vi "CurlingRobotforThrowingSTD.vi"() -> ()   [LabVIEW 2018]
uses:
  <vilib>/myRIO/Instrument Drivers/Onboard IO/DIO/typedefs/DIO Reference.ctl
  <vilib>/myRIO/Common/Instrument Driver Framework/Utilities/typedefs/myRIO Generic Hardware Reference.ctl
  <vilib>/myRIO/Common/Instrument Driver Framework/Utilities/typedefs/Hardware Version Enum.ctl
  <vilib>/myRIO/Common/Instrument Driver Framework/Utilities/typedefs/myRIO v1.0 Reference.ctl
  <vilib>/myRIO/Common/Instrument Driver Framework/Utilities/typedefs/Generic FPGA Reference.ctl
  <vilib>/myRIO/Common/Instrument Driver Framework/myRIO v1.0/DIO/typedefs/DIO Channels List.ctl
  <vilib>/myRIO/Common/Instrument Driver Framework/myRIO v1.0/DIO/typedefs/DIO Channels Enum.ctl
  <vilib>/userdefined/High Color/nirio_resource_hc.ctl
  <vilib>/myRIO/Instrument Drivers/Onboard IO/AO/typedefs/AO Reference.ctl
  <vilib>/myRIO/Common/Instrument Driver Framework/myRIO v1.0/AO/typedefs/AO Channels List.ctl
  <vilib>/myRIO/Common/Instrument Driver Framework/myRIO v1.0/AO/typedefs/AO Channels Enum.ctl
  <vilib>/myRIO/Common/Instrument Driver Framework/Utilities/typedefs/Analog Scaling Constants List.ctl
  <vilib>/myRIO/Common/Instrument Driver Framework/Utilities/typedefs/Analog Scaling Constants.ctl
  <vilib>/myRIO/Instrument Drivers/Onboard IO/I2C/typedefs/I2C User Configuration.ctl
  <vilib>/myRIO/Instrument Drivers/Onboard IO/I2C/typedefs/I2C Transfer Rate.ctl
  <vilib>/Platform/TimedLoop/XDataNode/timing_clust.ctl
  <vilib>/Platform/TimedLoop/XDataNode/nitl_modes.ctl
  <vilib>/Platform/TimedLoop/XDataNode/wakeup.ctl
  <vilib>/myRIO/Instrument Drivers/Onboard Devices/Accelerometer/typedefs/Accelerometer Reference.ctl
  <vilib>/myRIO/Common/Instrument Driver Framework/myRIO v1.0/Accelerometer/typedefs/Accelerometer Channels List.ctl
  <vilib>/myRIO/Common/Instrument Driver Framework/myRIO v1.0/Accelerometer/typedefs/Accelerometer Channels Enum.ctl
  <vilib>/myRIO/Common/Instrument Driver Framework/myRIO v1.0/Encoder/typedefs/Encoder Signal Mode.ctl
  <vilib>/myRIO/Instrument Drivers/Onboard IO/Encoder/typedefs/Encoder Reference.ctl
  <vilib>/myRIO/Common/Instrument Driver Framework/myRIO v1.0/Encoder/typedefs/Encoder Channels Enum.ctl
  <vilib>/myRIO/Common/Instrument Driver Framework/myRIO v1.0/Encoder/typedefs/Encoder Configuration v1.0.ctl
  <vilib>/myRIO/Common/Instrument Driver Framework/Utilities/vis/Is FPGA Ref Available.vi
  <vilib>/myRIO/Common/Instrument Driver Framework/myRIO v1.0/DIO/vis/myRIO v1.1 Open DIO.vi
  <vilib>/myRIO/Common/Instrument Driver Framework/myRIO v1.0/AO/vis/myRIO v1.1 Open AO.vi
  <vilib>/myRIO/Common/Instrument Driver Framework/myRIO v1.0/Accelerometer/vis/myRIO v1.1 Open Accelerometer.vi
  <vilib>/myRIO/Instrument Drivers/Onboard Devices/Accelerometer/vis/Read.vi
  <vilib>/myRIO/Common/Instrument Driver Framework/myRIO v1.0/Encoder/vis/myRIO v1.1 Open Encoder.vi
  <vilib>/myRIO/Instrument Drivers/Onboard IO/Encoder/vis/Read.vi
  <vilib>/myRIO/Common/Instrument Driver Framework/Utilities/vis/Validate Channels.vi
  <vilib>/myRIO/Common/Instrument Driver Framework/myRIO v1.0/DIO/vis/myRIO v1.0 Reserve DIO.vi
  <vilib>/myRIO/Common/Instrument Driver Framework/myRIO v1.0/AO/vis/myRIO v1.0 Reserve AO.vi
  <vilib>/myRIO/Common/Instrument Driver Framework/myRIO v1.0/Accelerometer/vis/myRIO v1.0 Reserve Accelerometer.vi
  <vilib>/myRIO/Common/Instrument Driver Framework/myRIO v1.0/I2C/vis/myRIO v1.1 Open I2C.vi
  <vilib>/myRIO/Common/Instrument Driver Framework/myRIO v1.0/Encoder/vis/myRIO v1.0 Reserve Encoder.vi
  <vilib>/myRIO/Common/Instrument Driver Framework/myRIO v1.0/UART/vis/myRIO v1.0 Close UART.vi
  <vilib>/myRIO/Common/Instrument Driver Framework/myRIO v1.0/Resource Manager/vis/myRIO v1.0 Reserve Channel List.vi
  <vilib>/myRIO/Common/Instrument Driver Framework/myRIO v1.0/DIO/vis/myRIO v1.0 Build MUX Configuration DIO.vi
  <vilib>/myRIO/Common/Instrument Driver Framework/myRIO v1.0/AO/vis/myRIO v1.0 Build MUX Configuration AO.vi
  <vilib>/myRIO/Common/Instrument Driver Framework/myRIO v1.0/Accelerometer/vis/myRIO v1.0 Build MUX Configuration Accelerometer.vi
  <vilib>/myRIO/Common/Instrument Driver Framework/myRIO v1.0/I2C/vis/myRIO v1.0 Reserve I2C.vi
  <vilib>/myRIO/Common/Instrument Driver Framework/myRIO v1.0/Encoder/vis/myRIO v1.0 Build MUX Configuration Encoder.vi
  <vilib>/myRIO/Common/Instrument Driver Framework/myRIO v1.0/Resource Manager/vis/myRIO v1.0 Reserve Channel.vi
  <vilib>/myRIO/Common/Instrument Driver Framework/myRIO v1.0/Resource Manager/vis/myRIO v1.0 Unreserve Channel.vi
  <vilib>/myRIO/Common/Instrument Driver Framework/myRIO v1.0/Resource Manager/vis/myRIO v1.0 Create Configuration List.vi
  <vilib>/myRIO/Common/Instrument Driver Framework/myRIO v1.0/I2C/vis/myRIO v1.0 Build MUX Configuration I2C.vi
  <vilib>/myRIO/Common/Instrument Driver Framework/myRIO v1.0/Resource Manager/vis/myRIO v1.0 Build Mutex Name.vi
  <vilib>/Instr/_visa.llb/VISA Configure Serial Port (Instr).vi
  <vilib>/Utility/VariantDataType/GetNumericInfo.vi
  <vilib>/Utility/error.llb/Error Cluster From Error Code.vi
  <vilib>/myRIO/Common/Instrument Driver Framework/myRIO v1.0/myRIO v1.1 Open.vi
  <vilib>/myRIO/Common/Instrument Driver Framework/Utilities/vis/IO Manager.vi
  <vilib>/myRIO/Common/Instrument Driver Framework/Utilities/vis/Configuration Manager.vi
  <vilib>/myRIO/Common/Instrument Driver Framework/myRIO v1.0/Resource Manager/vis/myRIO v1.0 Configure IO.vi
  <vilib>/myRIO/Common/Instrument Driver Framework/myRIO v1.0/myRIO v1.0 Close.vi
  <vilib>/myRIO/Common/Instrument Driver Framework/myRIO v1.0/DIO/vis/myRIO v1.0 Write DIO.vi
  <vilib>/myRIO/Common/Instrument Driver Framework/myRIO v1.0/AO/vis/myRIO v1.0 Get Scaling Constants AO.vi
  <vilib>/myRIO/Common/Instrument Driver Framework/myRIO v1.0/AO/vis/myRIO v1.0 Write AO.vi
  <vilib>/myRIO/Common/Instrument Driver Framework/myRIO v1.0/I2C/vis/myRIO v1.0 Configure I2C.vi
  <vilib>/myRIO/Common/Instrument Driver Framework/myRIO v1.0/I2C/vis/myRIO v1.0 Write I2C.vi
  <vilib>/myRIO/Common/Instrument Driver Framework/myRIO v1.0/Encoder/vis/myRIO v1.0 Configure Encoder.vi
  <vilib>/myRIO/Common/Instrument Driver Framework/myRIO v1.0/Encoder/vis/myRIO v1.0 Read Encoder.vi
  <vilib>/myRIO/Common/Instrument Driver Framework/myRIO v1.0/I2C/vis/myRIO v1.0 Read I2C.vi
  <vilib>/myRIO/Common/Instrument Driver Framework/Utilities/vis/FPGA Ref Manager.vi
  <vilib>/myRIO/Common/Instrument Driver Framework/myRIO v1.0/myRIO v1.0 Reset FPGA.vi
  <vilib>/myRIO/Common/Instrument Driver Framework/myRIO v1.0/IRQ/vis/myRIO v1.0 IRQ Info FGV.vi
  <vilib>/myRIO/Common/Instrument Driver Framework/myRIO v1.0/IRQ/vis/myRIO v1.0 Timer IRQ Info FGV.vi
  <vilib>/myRIO/Common/Instrument Driver Framework/myRIO v1.0/IRQ/vis/myRIO v1.0 ISR Agent.vi
  <vilib>/myRIO/Common/Instrument Driver Framework/myRIO v1.0/Accelerometer/vis/myRIO v1.0 Get Scaling Constant Accelerometer.vi
  <vilib>/myRIO/Common/Instrument Driver Framework/myRIO v1.0/Accelerometer/vis/myRIO v1.0 Read Accelerometer.vi
  <vilib>/myRIO/Express VI/Onboard IO/DO/DO Express VI.xnode
  <vilib>/myRIO/Instrument Drivers/Onboard IO/DIO/vis/myRIO DIO Open.xnode
  <vilib>/myRIO/Express VI/Onboard IO/AO/AO Express VI.xnode
  <vilib>/myRIO/Instrument Drivers/Onboard IO/AO/vis/myRIO AO Open.xnode
  <vilib>/Platform/TimedLoop/XDataNode/XDataNode.xnode
  <vilib>/myRIO/Express VI/Onboard IO/Encoder/Encoder Express VI.xnode
  <vilib>/myRIO/Instrument Drivers/Onboard IO/Encoder/vis/myRIO Encoder Open.xnode
  <vilib>/myRIO/Common/Instrument Driver Framework/myRIO v1.0/Encoder/typedefs/Encoder Count Direction Enum.ctl
  <vilib>/myRIO/Express VI/Onboard Devices/Accelerometer/Accelerometer Express VI.xnode
  <vilib>/myRIO/Instrument Drivers/Onboard Devices/Accelerometer/vis/myRIO Accelerometer Open.xnode
  <vilib>/Platform/TimedLoop/XDataNode/XDNodeRunTimeDep.lvlib
  <vilib>/myRIO/Instrument Drivers/Onboard IO/I2C/I2C.lvlib
  <vilib>/myRIO/Instrument Drivers/Utilities/Utilities.lvlib
  <vilib>/myRIO/Instrument Drivers/Onboard IO/Encoder/Encoder.lvlib
  <vilib>/myRIO/Instrument Drivers/Onboard IO/DIO/DIO.lvlib
  <vilib>/myRIO/Instrument Drivers/Onboard IO/AO/AO.lvlib
  <vilib>/myRIO/Instrument Drivers/Onboard Devices/Accelerometer/Accelerometer.lvlib
panel:
  out "DEn":bool
  out "StEn":bool
  out "RearEn":i16
  out "Readyon":bool
  out "YRRef":dbl
  out "YRRefOn":dbl
  out "RotFB":dbl
  out "RotFF":dbl
  out "IniSteerCmd":dbl=-0.08438764299664774
  in  "deg/Volt":dbl=2.8
  in  "SteerOri":dbl=391.05
  in  "StRefCut":dbl=1.0
  out "Tq_Steer":dbl=5.4e-323
  out "ori_phi":dbl(graph)=352.282379
  in  "SaveReset":bool
  in  "file create":bool
  out "File create":i32
  out "write":bool
  out "data innter":i32
  out "reset":bool
  out "Numeric Control":i32
  out "DriveMode":dbl(graph)=5.0
  out "PhiErr":dbl=-0.07207549693756998
  in  "LimStopErrVel":dbl=1.1
  in  "Cut_StopErr":dbl=3.0
  in  "KpStopError":dbl=10.0 format="%#_13g"
  in  "Ome_FB_Ratelimit(off)":bool=TRUE
  in  "Rear_scale":dbl=1.5 format="%#_13g"
  in  "FFOn":bool=TRUE
  in  "scale_Ang_steer/ 2":dbl=1.0 format="%#_13g"
  out "Tq_vel":cluster{dbl, dbl, "MinW":dbl}(graph)={-2.87e-322, -2.87e-322, "MinW"=2e-323} caption="CompareVel"
  in  "ShiftVelcrit":dbl=0.93 format="%#_13g"
  out "Ang":cluster{dbl, "y":dbl, dbl}(graph)
  out "AngError":dbl=2.6668637993124005
  out "tq":i32=5
  out "kvh":i32=501
  in  "No SRC(off)":bool=TRUE
  in  "Anti_wind":bool
  out "Wind_E":dbl
  in  "K_antiwind":dbl=0.5
  in  "criteria ang1":dbl=0.07
  in  "criteria ang2":dbl=2.0
  in  "ini_phi_2":dbl=5.0
  in  "ini_phi_1":dbl=1.5
  in  "DriveStart_manual":bool
  out "Driving":bool
  out "Ome_R":dbl=1.8e-322
  out "Ome_L":dbl=1.8e-322
  out "AngNowFB":dbl=-0.8036161356018248
  in  "scale_Ang_steer/":dbl=1.5 format="%#_13g"
  in  "Mode4_manual\n(get now ang)":bool
  in  "YR*_Off(manual)":bool=TRUE
  in  "From_SBC_DOB":bool
  in  "V*manualn":dbl=0.8
  in  "AutoSBCOn":bool=TRUE
  in  "Angle*_manual":dbl
  out "Time_int":i32=2781129
  in  "Steeing_Tq*_limit":dbl=5.0
  in  "YawConton":bool
  in  "Rear_DriveE":bool
  in  "Drive_Enable":bool
  in  "Rear_steerEnable":bool
  in  "Front enable":bool
  in  "Kt_longi":dbl=0.12
  in  "B_FF_R_wh":dbl=0.008
  in  "J_FF_R_wh":dbl=0.05
  in  "right wheel FF_cut 2":dbl=8.0
  in  "ylimit":dbl=0.2 format="%#_13g"
  out "Ome_ref":dbl
  in  "sigma_rate":dbl=0.0008 format="%#_13g"
  out "Ome_rear":dbl=-1.8e-322
  out "V+yS":dbl=2e-323
  out "VwRef":dbl=2e-323
  out "V+yV":dbl=2e-323
  out "y*(Ki+Kp)":dbl=-2.5e-323
  out "Ki_y":dbl
  out "Kp_y":dbl=-2.5e-323
  out "Vref":dbl
  in  "Vw*limitby_sigma":dbl=1.0 format="%#_13g"
  in  "Vel_treshold":dbl=0.6 format="%#_13g"
  in  "(1+y)_change":dbl=1.0 format="%#_13g"
  in  "Kp_V_cont 2":dbl=1.3
  in  "Ki_V_cont":dbl
  out "Sigmafor V+ySigma=Vw":dbl
  in  "Ki_wheel\nomega_cont":dbl
  in  "Kp_wheelomega_Cont":dbl=1.9
  out "Tq_cmd_R":dbl=-2.87e-322
  out "Tq_cmd_L":dbl=-2.87e-322
  in  "Tq limit[V]":dbl=10.0
  out "Vel_Robot":dbl=2e-323
  in  "Wheelvel_ratelimit cut":dbl=20.0
  in  "wheelV_ratelimit":dbl=0.001
  out "th_steer":dbl=0.11066568835903608
  in  "Enc_steer":bool
  out "l_rear":dbl=0.1917516891011395
  in  "Enc_set 0":bool
  out "l_L 2":dbl=0.1944940376883356
  out "l_R 2":dbl=0.14254976665663685
  in  "Tq_stop":dbl=-3.0 format="%#_13g"
  out "back stop":bool
  out "back driving act":bool
  in  "Desire back dist":dbl=2.5
  out "Back driving time":dbl=47.62300000000005
  in  "nowphi_in":dbl
  out "dist_avr":dbl=0.14254976665663685
  in  "ref_LFP_cut":dbl=10.0
  in  "ang_compensate":dbl
  in  "Bm_rot FF":dbl=0.1
  in  "Jm_rotFF":dbl=0.1
  in  "gyro scale":dbl=0.3
  out "delta_ang_memo":dbl
  out "fine_tunning":sgl=1.0
  out "nowphi":dbl
  in  "Stop":bool
  out "Data":string
  out "*(타입 *) &x":T1={"header"=43520, "type"=10, "data0"=5.0, "data1"=390.6329}
  out "driveONoFF":dbl format="%#_13g"
  out "DriveMODE":dbl=5.0 format="%#_13g"
  out "SteerAng":dbl=390.6329040527344 format="%#_13g"
  out "Target_V":dbl=2.3801119327545166 format="%#_13g"
  out "angle":dbl=2.4951019287109375 format="%#_13g"
  in  "Server Closed":string="The server VI closed the connection."
  in  "Stop Button":bool
  in  "phi_target":dbl
  in  "Kt_rot":dbl=0.093 format="%#_13g"
  out "AngNowCmd":dbl=-0.8756916325393947
  in  "PD_cut_rot 2":dbl=10.0
  in  "Kp_rot 3":dbl=0.0005
  in  "Kd_rot 4":dbl=0.0001
  out "ang_bias remover":dbl=0.8036191995518251
  out "Abs angle or gyro":dbl=352.282379
  in  "abs gy stop Button":bool
  in  "ratelimit band":dbl=0.0009
  in  "ratelimit cut":dbl=30.0
  in  "yaw_ratelimit":dbl=0.003
  out "time_now":u32=3177835
  out "Tq ang in":dbl=8e-323
  out "DOB FB":dbl=-0.0
  out "GyroFB":dbl
  in  "gy_offset_remover cutoff":dbl=0.05
  in  "Kd_rot 3":dbl=0.001
  in  "Kp_rot 2":dbl=0.005
  in  "PD_cut_rot":dbl=13.0
  in  "FF_cut":dbl=5.0
  in  "DOB_FB_cut":dbl=13.0
  in  "Bm_rot":dbl=0.1
  in  "Jm_rot":dbl=0.15
  in  "Vel_cut":dbl=25.0
  out "Z rate":i16=253
  in  "[main loop]":bool
  out "Tq_cmd_Rear":dbl=2.57e-322
  # "manual Driving"
  # "manual Driving and Auto from SBC selection"
  # "Auto Driving"
  # "Initial"
  # "Yaw ref"
  # "longi vel cmd"
  # "Output"
  # "wheel_vel_ratelimeter"
  # "Longi vel control"
  # "SRC"
  # "Anti-wind"
  # "Yaw control"
  # "Yaw  rate control"
  # "Dimension values"
  # "Yaw  rate control"
  # "Auto back"
  # "Fine turnning"
  # "anti windup"
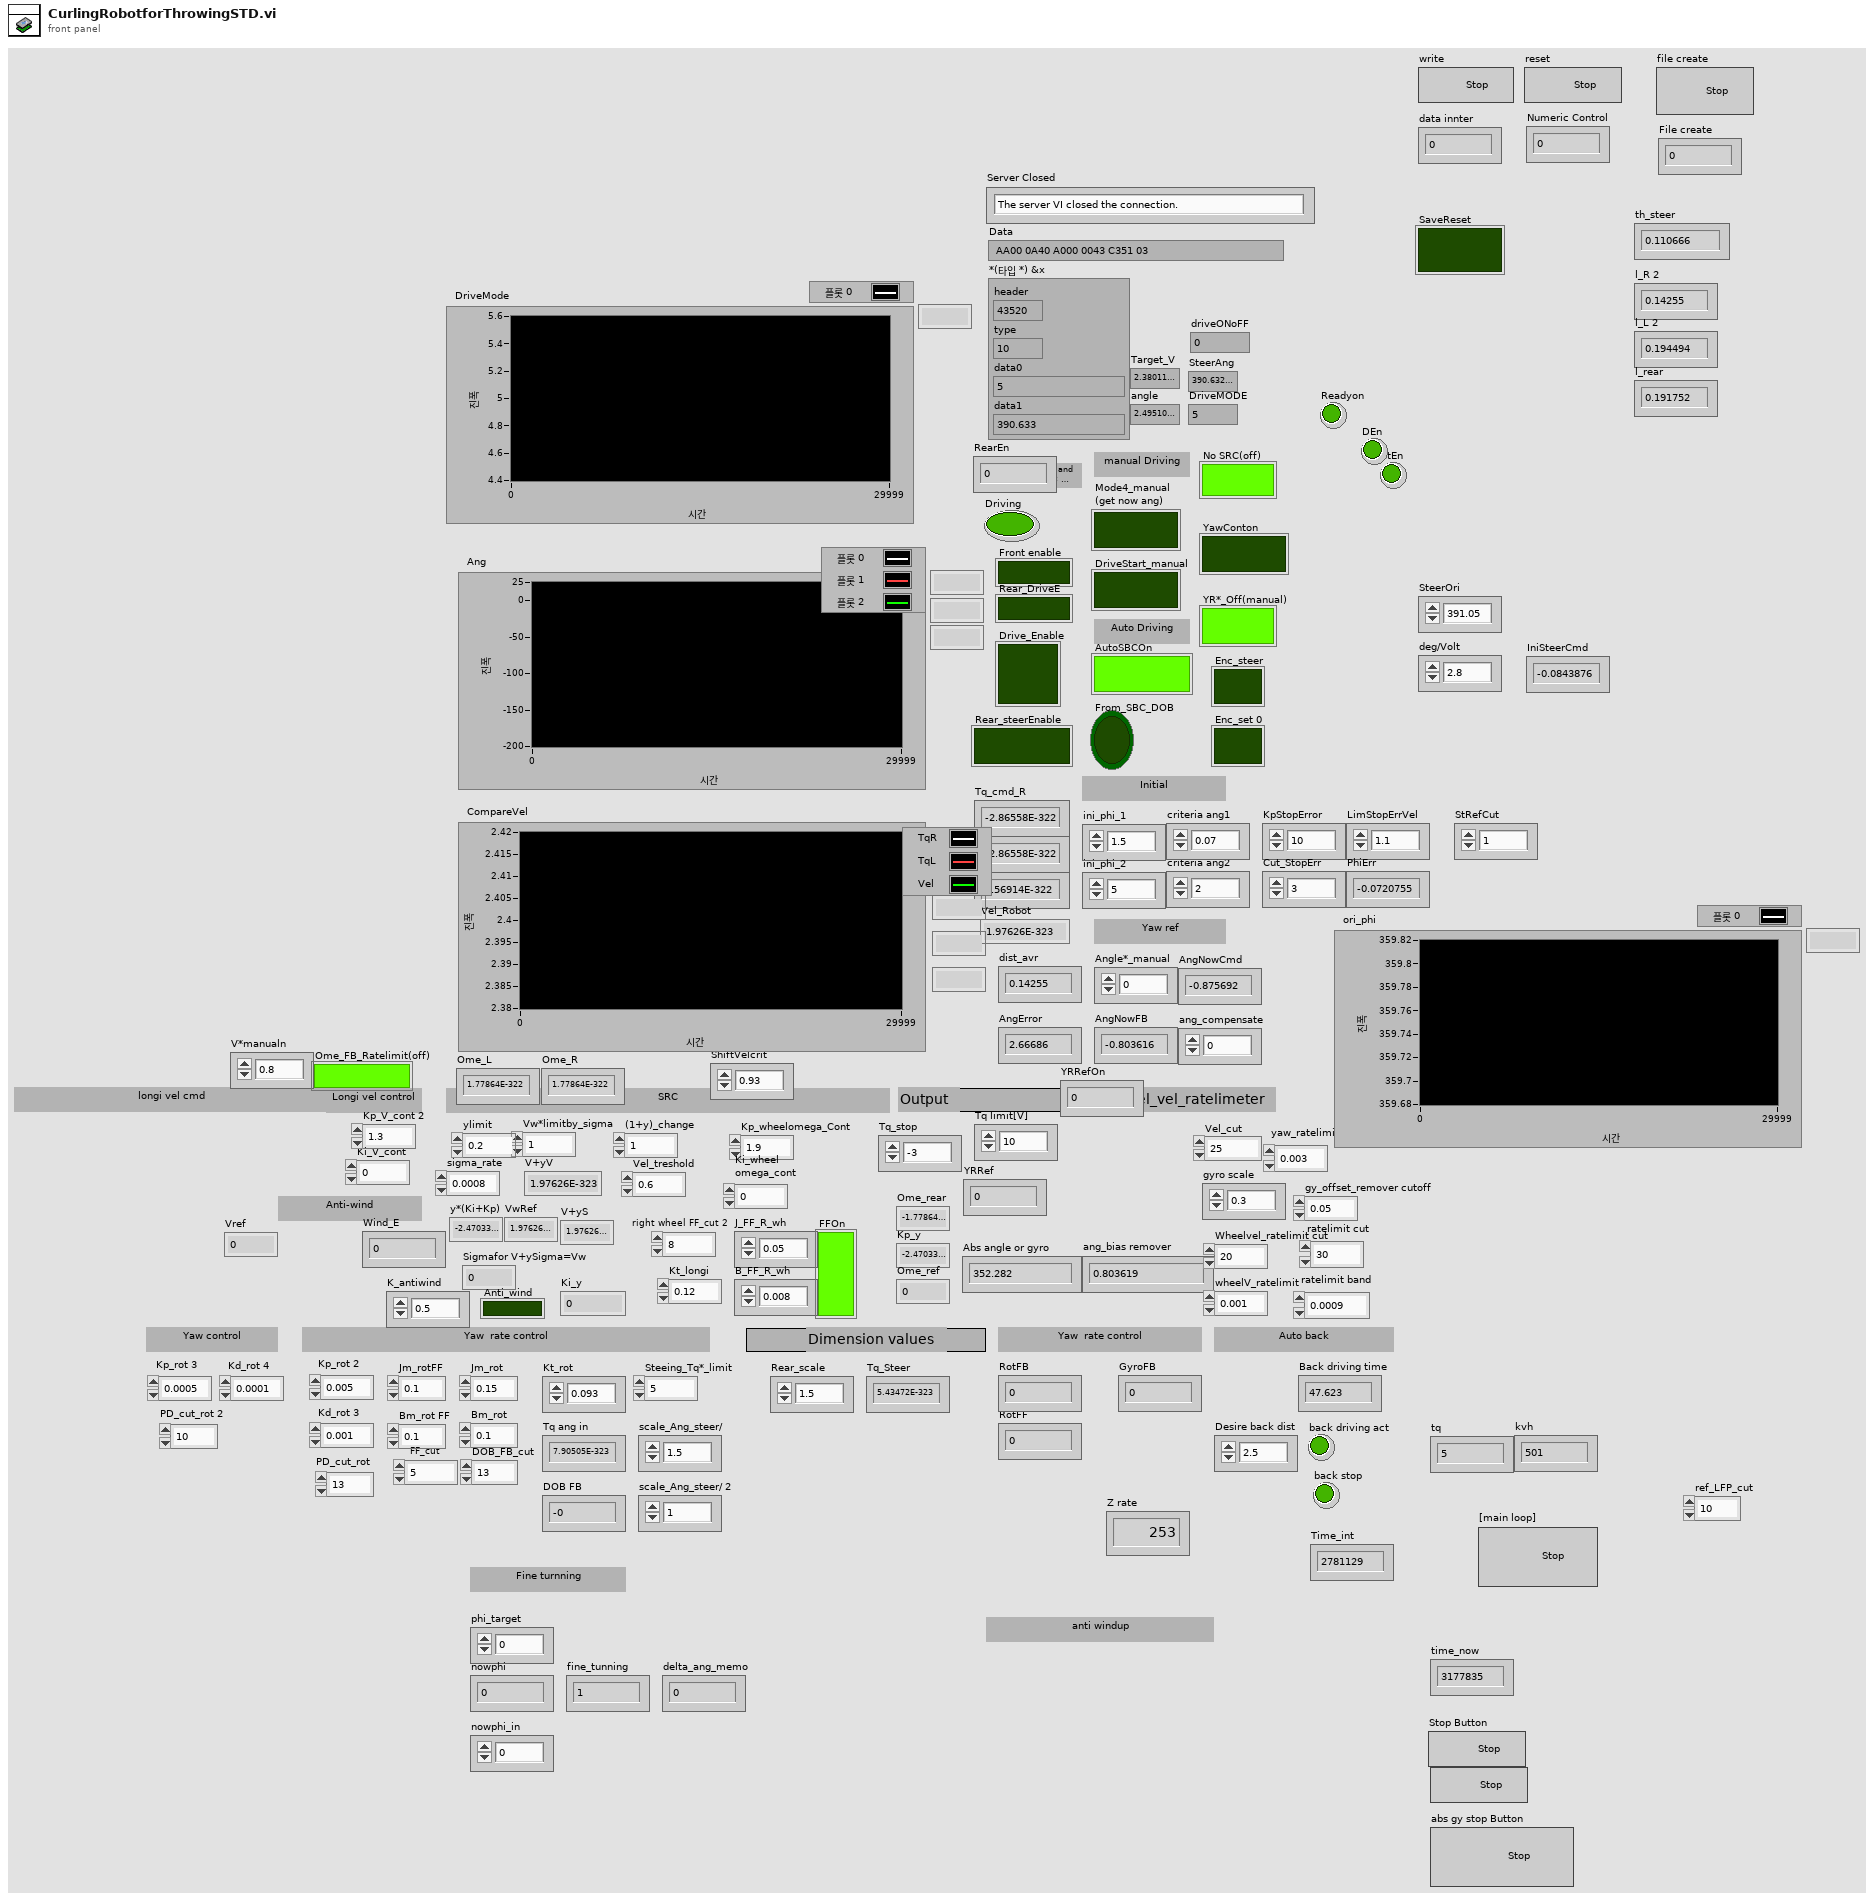
[diagram p1: front panel]
types:
  T1 = cluster{"header":u16, "type":u8, "data0":sgl, "data1":sgl}
  T2 = typedef "DIO.lvlib/DIO Reference.ctl" = cluster{"myRIO Reference":T3, "DIO Channels List":T7}
  T3 = typedef "myRIO Generic Hardware Reference.ctl" = cluster{"myRIO Model":T4, "myRIO Hardware Reference":T5}
  T4 = typedef "Hardware Version Enum.ctl" = enum16{"Unknown", "myRIO-1900", "myRIO-1950", "roboRIO", "NI ELVIS RIO CM", "ELVIS III"}
  T5 = typedef "myRIO v1.0 Reference.ctl" = cluster{"Generic FPGA Reference":T6, "Allow multiple opens":bool}
  T6 = typedef "Generic FPGA Reference.ctl" = refnum<k20>
  T7 = typedef "DIO Channels List.ctl" = T8[]
  T8 = typedef "DIO Channels Enum.ctl" = enum16{"Not Connected", "C/DIO0", "C/DIO1", "C/DIO2", "C/DIO3", "C/DIO4", "C/DIO5", "C/DIO6", "C/DIO7", "A/DIO0", "A/DIO1", "A/DIO2", "A/DIO3", "A/DIO4", "A/DIO5", "A/DIO6", "A/DIO7", "A/DIO8", "A/DIO9", "A/DIO10", "A/DIO11", "A/DIO12", "A/DIO13", "A/DIO14", "A/DIO15", "A/DIO16", "A/DIO17", "A/DIO18", "A/DIO19", "B/DIO0", "B/DIO1", "B/DIO2", "B/DIO3", "B/DIO4", "B/DIO5", "B/DIO6", "B/DIO7", "B/DIO8", "B/DIO9", "B/DIO10", "B/DIO11", "B/DIO12", "B/DIO13", "B/DIO14", "B/DIO15", "B/DIO16", "B/DIO17", "B/DIO18", "B/DIO19", "LED0", "LED1", "LED2", "LED3", "Button0", "DIO/DIO0", "DIO/DIO1", "DIO/DIO2", "DIO/DIO3", "DIO/DIO4", "DIO/DIO5", "DIO/DIO6", "DIO/DIO7", "DIO/DIO8", "DIO/DIO9", "SPI/CS0", "SPI/CS1", "SPI/CS2", "SPI/CS3", "LED RADIO (Green)", "LED RADIO (Red)", "LED COMM (Green)", "LED COMM (Red)", "LED MODE (Green)", "LED MODE (Red)"}
  T9 = typedef "nirio_resource_hc.ctl" = tag
  T10 = typedef "AO.lvlib/AO Reference.ctl" = cluster{"myRIO Reference":T3, "AO Channel List":T11, "AO Scaling Constant List":T13}
  T11 = typedef "AO Channels List.ctl" = T12[]
  T12 = typedef "AO Channels Enum.ctl" = enum16{"Not Connected", "AudioOut/Left", "AudioOut/Right", "C/AO0", "C/AO1", "A/AO0", "A/AO1", "B/AO0", "B/AO1"}
  T13 = typedef "Analog Scaling Constants List.ctl" = T14[]
  T14 = typedef "Analog Scaling Constants.ctl" = cluster{"LSB Weight (Volts)":dbl, "Offset (Volts)":dbl, "Signed?":bool}
  T15 = enum16{"open", "replace", "create", "open or create", "replace or create", "replace or create with confirmation"}
  T16 = typedef "Accelerometer.lvlib/Accelerometer Reference.ctl" = cluster{"myRIO Reference":T3, "Accelerometer Channels List":T17, "LSB Weight":dbl}
  T17 = typedef "Accelerometer Channels List.ctl" = T18[]
  T18 = typedef "Accelerometer Channels Enum.ctl" = enum16{"Not Connected", "X-Axis", "Y-Axis", "Z-Axis"}
  T19 = typedef "Encoder.lvlib/Encoder Reference.ctl" = cluster{"myRIO Reference":T3, "Encoder Channels Enum":T20}
  T20 = typedef "Encoder Channels Enum.ctl" = enum16{"Not Connected", "C/ENC0", "C/ENC1", "A/ENC", "A/ENC0", "A/ENC1", "A/ENC2", "A/ENC3", "A/ENC4", "A/ENC5", "A/ENC6", "A/ENC7", "A/ENC8", "A/ENC9", "B/ENC", "B/ENC0", "B/ENC1", "B/ENC2", "B/ENC3", "B/ENC4", "B/ENC5", "B/ENC6", "B/ENC7", "B/ENC8", "B/ENC9", "DIO/ENC0", "DIO/ENC1", "DIO/ENC2", "DIO/ENC3", "DIO/ENC4"}
  T21 = typedef "Encoder Signal Mode.ctl" = enum16{"Quadrature phase signal", "Step and direction signal"}
  T22 = typedef "XDNodeRunTimeDep.lvlib/timing_clust.ctl" = cluster{"Expected End [f-1]":u64, "Actual End [f-1]":u64, "Finished Late? [f-1]":bool, "Expected End [i-1]":u64, "Actual End [i-1]":u64, "Finished Late? [i-1]":bool, "Expected Start [i]":u64, "Actual Start [i]":u64, "Expected Start [f]":u64, "Actual Start [f]":u64, "Source Name":string, "Structure Name":string, "Period":i64, "Deadline":i64, "Offset":i64, "Start":i64, "Priority":i32, "Timeout":i32, "Mode":T23, "Wakeup Reason":T24, "Error":errorcluster, "Source Type":string, "Secondary Source Type":string, "Global End Time":u64, "Global Start Time":u64, "Frame Duration":u64, "Iteration Duration":u64, "Assigned CPU":i32, "I/O Scan Engine Mode":u32}
  T23 = typedef "XDNodeRunTimeDep.lvlib/nitl_modes.ctl" = enum32{"No Change", "Process missed periods, maintain original phase", "Discard missed periods, maintain original phase", "Process missed periods, ignore original phase", "Discard missed periods, ignore original phase"}
  T24 = typedef "XDNodeRunTimeDep.lvlib/wakeup.ctl" = enum32{"Normal", "Aborted", "Asynchronous wakeup", "Timing source error", "Timed loop error", "Timeout"}
  T25 = cluster{"baud rate (9600)":u32, "data bits (8)":u16, "parity (0:none)":enum16{"None", "Odd", "Even", "Mark", "Space"}, "stop bits (10: 1 bit)":u16, "flow control (0:none)":u16, "termination char\n(0xA = '\\n' = LF) ":u8, "Enable Termination\nChar (T)":bool, "timeout (10sec)":u32}
  T26 = typedef "I2C.lvlib/I2C User Configuration.ctl" = cluster{"I2C Transfer Rate":T27}
  T27 = typedef "I2C.lvlib/I2C Transfer Rate.ctl" = enum16{"Standard mode (100 kbps)", "Fast mode (400 kbps)"}
  T28 = typedef "I2C.lvlib/I2C Reference.ctl" = cluster{"myRIO Reference":T3, "I2C Channels Enum":T29, "I2C Configuration":T30}
  T29 = typedef "I2C Channels Enum.ctl" = enum16{"Not Connected", "A/I2C", "B/I2C", "I2C/I2C"}
  T30 = typedef "I2C.lvlib/I2C Configuration.ctl" = cluster{"I2C Transfer Rate":T27}
  T31 = cluster{"l_rear":dbl, "Vref":dbl, "Vel_Robot":dbl, "Ome_ref":dbl, "Ome_R":dbl, "Ome_L":dbl, "VwRef":dbl, "V+yV":dbl, "V+yS":dbl, "Ki_y":dbl, "Kp_y":dbl, "nowphi":dbl, "angle":dbl, "AngNowCmd":dbl, "AngNowFB":dbl, "delta_ang_memo":dbl, "DriveMode":dbl, "X-Axis":dbl, "Y-Axis":dbl, "Tq_cmd_R":dbl, "Tq_cmd_L":dbl, "Tq_cmd_Rear":dbl, "Tq_Steer":dbl, "th_steer":dbl, "SteerAng":dbl, "YRRefOn":dbl, "YRRef":dbl, "DOB FB":dbl, "RotFF":dbl, "RotFB":dbl, "ang_bias remover":dbl, dbl, dbl, dbl}
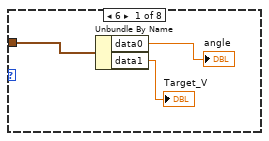
[diagram p6: hidden frame]
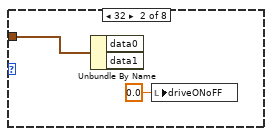
[diagram p7: hidden frame]
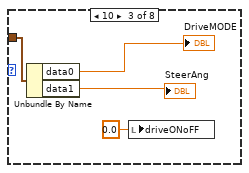
[diagram p8: hidden frame]
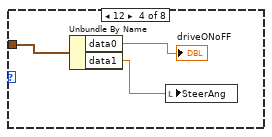
[diagram p9: hidden frame]
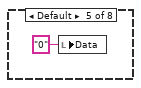
[diagram p10: hidden frame]
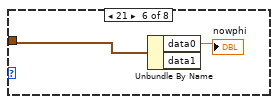
[diagram p11: hidden frame]
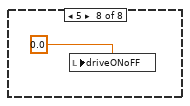
[diagram p12: hidden frame]
diagram:
  n1 = flat-sequence {
    frame #0 {
      w11 = T25 {"baud rate (9600)"=38400, "data bits (8)"=8, "parity (0:none)"=enum."None", "stop bits (10: 1 bit)"=10, "flow control (0:none)"=0, "termination char\n(0xA = '\\n' = LF) "=10, "Enable Termination\nChar (T)"=TRUE, "timeout (10sec)"=10000}  # VISA Configuration
      w12 = refnum<visa-resource-name> "ASRL1::INSTR"  # VISA resource name in
      n2 = Unbundle By Name(w11) -> ("Enable Termination\nChar (T)"=w10:bool, "termination char\n(0xA = '\\n' = LF)"=w9:u8, "timeout (10sec)"=w8:u32, "baud rate (9600)"=w3:u32, "data bits (8)"=w4:u16, "parity (0:none)"=w5:enum16{"None", "Odd", "Even", "Mark", "Space"}, "stop bits (10: 1 bit)"=w6:u16, "flow control (0:none)"=w7:u16)
      n3 = call-poly "VISA Configure Serial Port"("VISA resource name"=w12, "timeout (10sec)"=w8, "termination char\n(0xA = '\\n' = LF)"=w9, "Enable Termination\nChar (T)"=w10, "baud rate (9600)"=w3, "data bits (8)"=w4, "parity (0:none)"=w5, "stop bits (10: 1 bit)"=w6, "flow control (0:none)"=w7) -> ("VISA resource name out"=w2:refnum<visa-resource-name>, "error out"=w1:errorcluster)  [unwired: 5 in]
      n4 = while {
        tunnel: w2 -> [w105]
        tunnel: w1 -> [w104]
        tunnel: [w118] -> _
        i -> [w108]
        stop <- w102 stop-if-true
        w103 = 5.0  # y
        w119 = u32 10  # ms 배수
        n5 = Wait Until Next ms Multiple(millisecond multiple=w119) -> ()  [unwired: 1 out]
        n6 = Divide(x=w108, y=100) -> (x/y=w101:dbl)
        n7 = Greater?(x=w101, y=1.0) -> (0:w113:bool)
        n8 = Greater?(x=w101, y=3.0) -> (0:w110:bool)
        n9 = Greater?(x=w101, y=w103) -> (0:w102:bool)
        n10 = Less?(x=w101, y=2.0) -> (x < y?=w112:bool)
        n11 = Less?(x=w101, y=4.0) -> (x < y?=w109:bool)
        n12 = And(x=w110, y=w109) -> (x .and. y?=w106:bool)
        n13 = And(x=w113, y=w112) -> (x .and. y?=w107:bool)
        n14 = case shown="참" w107 {
          tunnel: w105 -> [_ w129]
          tunnel: w104 -> [w125 w128]
          tunnel: [w125 w127] -> w118
          frame False {
          }
          frame True {
            w126 = "Z"  # 명령 선택
            n15 = VISA Write(VISA resource name=w129, write buffer=w126, error in (no error)=w128) -> (error out=w127:errorcluster)  [unwired: 2 out]
          }
        }
        n16 = case shown="참" w106 {
          tunnel: w105 -> [_ w124]
          tunnel: w104 -> [w120 w123]
          tunnel: [w120 w122] -> _
          frame False {
          }
          frame True {
            w121 = "P"  # 명령 선택
            n17 = VISA Write(VISA resource name=w124, write buffer=w121, error in (no error)=w123) -> (error out=w122:errorcluster)  [unwired: 2 out]
          }
        }
        "kvh" <- w108
      }
      n18 = while {
        i -> [w16]
        stop <- w25 stop-if-true
        w22 = 1.5 ("C/AO0 (AO0)")
        w26 = 5.0  # y
        n19 = Divide(x=w16, y=10) -> (x/y=w14:dbl)
        "tq" <- w14
        n20 = Wait Until Next ms Multiple(millisecond multiple=u32 100 ("ms 배수")) -> ()  [unwired: 1 out]
        n21 = Greater?(x=w14, y=w26) -> (0:w25:bool)
        n22 = Negate(x=w22) -> (-x=w21:dbl)
        n23 = Greater?(x=w14, y=2.5) -> (0:w20:bool)
        n24 = Select(t=w21, s=w20, f=w22) -> (s? t:f=w23:dbl)
        n25 = xnode "Digital output (1 sample)"("C/DIO5 (DIO5)"=TRUE, "C/DIO7 (DIO7)"=FALSE) -> ()  [unwired: 1 in, 1 out]
        n26 = Negate(x=w23) -> (-x=w19:dbl)
        n27 = xnode "Analog output (1 sample) 2"("C/AO0 (AO0)"=w23, "C/AO1 (AO1)"=w19) -> ()  [unwired: 1 in, 1 out]
      }
    }
    frame #1 {
      w133 = T25 {"baud rate (9600)"=38400, "data bits (8)"=8, "parity (0:none)"=enum."None", "stop bits (10: 1 bit)"=10, "flow control (0:none)"=0, "termination char\n(0xA = '\\n' = LF) "=10, "Enable Termination\nChar (T)"=TRUE, "timeout (10sec)"=10000}  # VISA Configuration
      w132 = refnum<visa-resource-name> "ASRL1::INSTR"  # VISA resource name in
      w149 = T26 {"I2C Transfer Rate"=enum."Fast mode (400 kbps)"}  # I2C bus speed
      w148 = tag "A/I2C"  # I2C channel
      w155 = u8 105  # PmodGYRO address
      # "Integrate rate to obtain position"
      # "Enable INT1 & \"data ready\" interrupt on INT2 pin"
      # "CTRL_REG3"
      # "Select HPF cutoff frequency"
      # "CTRL_REG2"
      # "Output select for LPF/HPF (both bypassed)"
      # "CTRL_REG5"
      # "Initialize device"
      # "Select data rate and enable measurements"
      # "Z-axis HI threshold"
      # "Enable interrupt on Z greater than HI threshold"
      # "CTRL_REG1"
      # "INT1_THS_ZH"
      # "INT1_CFG"
      # "Full scale setting = 100 dps"
      # "CTRL_REG4"
      # "register / data"
      n28 = while {
        stop <- "Stop Button" stop-if-true
        w163 = u16 10200  # port
        w162 = "172.22.11.1"  # address
        n29 = TCP Open Connection(address=w162, remote port or service name=w163) -> (connection ID=w158:refnum<k5>, error out=w157:errorcluster)  [unwired: 3 in]
        n30 = while {
          tunnel: w157 -> [w184]
          tunnel: w158 -> [w185]
          tunnel: [w178] -> w164
          tunnel: [w177] -> w165
          stop <- w181 stop-if-true
          w183 = 11  # bytes to read
          # "TCP Client Loop"
          n31 = Wait Until Next ms Multiple(millisecond multiple=u32 1) -> ()  [unwired: 1 out]
          n32 = TCP Read(connection ID=w185, bytes to read=w183, error in (no error)=w184, 9:-1 ("timeout ms (25000)")) -> (connection ID out=w178:refnum<k5>, data out=w179:string, error out=w177:errorcluster)  [unwired: 1 in]
          "Data" <- w179
          n33 = Or(x=w177, y="Stop") -> (x .or. y?=w181:bool)
          n34 = Type Cast(type=T1 {"header"=0, "type"=0, "data0"=0.0, "data1"=0.0}, x=w179) -> (*(type *) &x=w174:T1)
          "*(타입 *) &x" <- w174
          n35 = Unbundle By Name(w174) -> ("type"=w176:u8)
          n36 = case shown="22" w176 {
            tunnel: w174 -> [w188 w190 w193 w196 _ w200 w202 _]
            frame 6 {
              n37 = Unbundle By Name(w188) -> ("data0"=→"angle":sgl, "data1"=→"Target_V":sgl)
            }
            frame 32 {
              n38 = Unbundle By Name(w190) -> ()  [unwired: 2 out]
              n39 = local write "driveONoFF"(0.0 ("DriveMODE")) -> ()
            }
            frame 10 {
              n40 = Unbundle By Name(w193) -> ("data0"=→"DriveMODE":sgl, "data1"=→"SteerAng":sgl)
              n41 = local write "driveONoFF"(0.0 ("driveONoFF")) -> ()
            }
            frame 12 {
              n42 = Unbundle By Name(w196) -> ("data0"=→"driveONoFF":sgl, "data1"=w195:sgl)
              n43 = local write "SteerAng"(w195) -> ()
            }
            frame Default {
              n44 = local write "Data"("0" ("Data")) -> ()
            }
            frame 21 {
              n45 = Unbundle By Name(w200) -> ("data0"=→"nowphi":sgl)  [unwired: 1 out]
            }
            frame 22 {
              n46 = Unbundle By Name(w202) -> ("data0"=→"fine_tunning":sgl)  [unwired: 1 out]
            }
            frame 5 {
              n47 = local write "driveONoFF"(0.0 ("DriveMODE")) -> ()
            }
          }
        }
        n48 = TCP Close Connection(connection ID=w164, error in (no error)=w165) -> (error out=w160:errorcluster)  [unwired: 1 in, 1 out]
        n49 = case shown="에러" w160 {
          selector: w160 -> [w166 w168]
          tunnel: [w166 w167] -> w161
          frame No Error {
          }
          frame Error {
            n50 = Unbundle By Name(w168) -> ("code"=w169:i32)
            n51 = case shown="62, 64, 66" w169 {
              tunnel: w168 -> [w170 _]
              tunnel: [w170 w172] -> w167
              frame Default {
              }
              frame 62, 64, 66 {
                w172 = errorcluster {"status"=FALSE, "code"=0, "source"=""}  # No error
                n52 = One Button Dialog(message="Server Closed") -> ()  [unwired: 1 in, 1 out]
              }
            }
          }
        }
        n53 = call <vilib>:"Simple Error Handler.vi"("error in (no error)"=w161) -> ()  [unwired: 4 in, 5 out]
      }
      n54 = Unbundle By Name(w133) -> ("Enable Termination\nChar (T)"=w136:bool, "termination char\n(0xA = '\\n' = LF)"=w137:u8, "timeout (10sec)"=w138:u32, "baud rate (9600)"=w143:u32, "data bits (8)"=w142:u16, "parity (0:none)"=w141:enum16{"None", "Odd", "Even", "Mark", "Space"}, "stop bits (10: 1 bit)"=w140:u16, "flow control (0:none)"=w139:u16)
      n55 = call <vilib>:"Open.vi"("Channel Name"=w148) -> ("error out"=w151:errorcluster, "I2C Ref Out"=w150:T28)  [unwired: 9 in]
      n56 = call <vilib>:"Configure.vi"("error in (no error)"=w151, "I2C User Configuration"=w149, "I2C Ref In"=w150) -> ("error out"=w154:errorcluster, "I2C Ref Out"=w153:T28)  [unwired: 7 in]
      n57 = call-poly "VISA Configure Serial Port"("VISA resource name"=w132, "timeout (10sec)"=w138, "termination char\n(0xA = '\\n' = LF)"=w137, "Enable Termination\nChar (T)"=w136, "baud rate (9600)"=w143, "data bits (8)"=w142, "parity (0:none)"=w141, "stop bits (10: 1 bit)"=w140, "flow control (0:none)"=w139) -> ("VISA resource name out"=w134:refnum<visa-resource-name>, "error out"=w135:errorcluster)  [unwired: 5 in]
      n58 = while {
        tunnel: w134 -> [w322]
        tunnel: w135 -> [w321]
        stop <- "abs gy stop Button" stop-if-true
        w319 = u32 256  # 바이트 카운트
        n59 = property class="Instr" props=["Serial Settings:Number of Bytes at Serial Port"](reference=w322) -> (reference out=w320:refnum<visa-resource-name>)  [unwired: 1 in, 2 out]
        n60 = call <vilib>:"Space Constant.vi"() -> ("String"=w315:string)
        n61 = VISA Read(VISA resource name=w320, byte count=w319, error in (no error)=w321) -> (read buffer=w318:string)  [unwired: 3 out]
        n62 = call <vilib>:"Trim Whitespace.vi"("string"=w318) -> ("trimmed string"=w317:string)  [unwired: 1 in]
        n63 = Match Pattern(string=w317, regular expression=w315) -> (before substring=w316:string)  [unwired: 1 in, 3 out]
        n64 = call <vilib>:"Trim Whitespace.vi"("string"=w316) -> ("trimmed string"=w314:string)  [unwired: 1 in]
        n65 = Fract/Exp String To Number(string=w314) -> (number=→"Abs angle or gyro":dbl)  [unwired: 3 in, 1 out]
        n66 = Wait Until Next ms Multiple(millisecond multiple=u32 1 ("ms 배수")) -> ()  [unwired: 1 out]
      }
      n67 = for {
        tunnel: [w1515] -> w145
        tunnel: [w1514] -> w144
        tunnel: [w1510] -> w146
        tunnel: u8[][] [[34, 136], [35, 0], [48, 32], [54, 80], [36, 0], [33, 9], [32, 15]] ("Bytes to Write") -> [w1513] mode=indexing
        tunnel: w153 -> [w1512]
        tunnel: w154 -> [w1511]
        tunnel: w155 -> [w1510]
        n68 = call <vilib>:"Write.vi"("error in (no error)"=w1511, "Bytes to Write"=w1513, "Slave Address (7-bit)"=w1510, "I2C Ref In"=w1512) -> ("error out"=w1515:errorcluster, "I2C Ref Out"=w1514:T28)  [unwired: 6 in]
      }
      n69 = node-c288() -> (w131:T22)  [unwired: 4 in]
      n70 = timed-loop {
        timing: w131 -> [_]
        timing-out: [_] -> w130
        tunnel: w144 -> [w1004]
        tunnel: w145 -> [w1003]
        tunnel: [w1001] -> w147
        tunnel: w146 -> [w1002]
        i -> [w700]
        stop <- "[main loop]" stop-if-true
        w604 = 10.0 ("y")
        w366 = 0.0 ("f")
        w408 = 0.5 ("y")
        w347 = 13.0 ("y")
        w682 = 0.0 ("f")
        w763 = 0.0 ("y0")
        w765 = 0.001 ("input variable")
        w832 = 3.0 ("y")
        w946 = 0.0
        w878 = 0.0
        w1048 = 0.0
        w1109 = 0.001 ("input variable")
        # "SteerIniSwitch"
        # "SteerCmdSwitch"
        # "Enable"
        # "steer rotate to fine tunning"
        # "steer rotate to origin"
        # "EnableSteer"
        # "10-1 Steer Enable Off"
        # "To get Steering Initializing"
        # "No anti slip"
        # "after acceleration vel"
        # "waiting for braking time"
        # "rear initialize on"
        # "autoback drive on"
        # "autoback front"
        # "Back driving vel"
        # "Vel robot"
        # "SteerRefLPF to initialization"
        # "Saturation"
        # "rear velocity to initialization"
        # "move rear until 0phierror\n become small or time"
        # "SteerCmdChange"
        # "Saturation"
        # "To get time to rotate robot to target angle"
        # "To prevent rotate when vel=0"
        # "DOB on or off"
        # "Anti wind up for y"
        # "when Braking On -->off"
        # "SRC on or Off"
        # "V_robot"
        # "V_robot"
        # "Rear wheel FF"
        # "Left wheel FF"
        # "Right wheel FF"
        # "y"
        # "V+y*Sigma"
        # "Simga"
        # "y"
        # "Criteria_Vx"
        # "Select manual Omega"
        # "Select manual Tq"
        # "Vw_PI controller 3wheels"
        # "T_R*"
        # "Offset remove for KVH Yaw sensor"
        # "Rbot velocity Estimation\n1) put in rate limit each wheel.\n2) pick up mim wheelvel among 3-wheel.\n3) KKF with acceleration"
        # "rated limiter"
        # "rated limiter"
        # "rated limiter"
        # "cnt/rev19bit"
        # "Data saving"
        # "Time derivative of enc to gel wheel vel"
        # "Wheel encoder gear ratio, encoder"
        # "gear ratio"
        # "gear ratio"
        # "Stopping Time"
        # "Stopping Timerange\n0.5+0.001"
        # "Stopping negative Tq"
        # "Select joystick& autorun"
        # "Joiski or autoback"
        # "Back driving  Distance limit"
        # "For back driving"
        # "Back driving on time"
        # "Auto back time increase Reset"
        # "when stand by mode get distance"
        # "wherthere dist great than 6 miter"
        # "Auto back distance memory"
        # "Starting angle driving timinng"
        # "Tq rot in"
        # "Indicate"
        # "Reset ENC"
        # "contain phi"
        # "phi_FB"
        # "calculate delta x,y,phi"
        # "fine turnning for set origin"
        # "To remove 360.6~~"
        # "angle limit +-180"
        # "To get origine angle"
        # "YR_ref"
        # "Read three 16-bit gyroscope values:\nWrite the address of the first register with MSB set to enable auto-indexing and then read six bytes"
        # "Format the six bytes into three 16-bit integers"
        # "calculatefixed offset"
        # "Rate limiter"
        # "rated limiter"
        # "Stop release to SBC through TCP/IP"
        # "when button start and stop within dive time automatly"
        # "Tq rot in"
        # "Gyro FB"
        # "Tq rot in"
        # "FF"
        # "Gyro FB"
        # "YMObser"
        # "YMO controller"
        # "Tq_Right"
        # "Rot PD  controller"
        n71 = node-c288() -> ()  [unwired: 1 in, 1 out]
        n72 = local read "ang_bias remover"() -> (w934:dbl)
        n73 = formula code="float phi;\nif (sensor > 180 && sensor <= 360)\nphi = sensor-360;\nelse\nphi = sensor;"("sensor"=w934) -> ("phi"=w935:dbl)
        n74 = local read "angle"() -> (w642:dbl)
        n75 = local read "DriveMODE"() -> (w953:dbl)
        n76 = Select(t=w642, s="AutoSBCOn", f="Angle*_manual") -> (s? t:f=w639:dbl)
        n77 = Equal?(x=w953, y=4.0) -> (x = y?=w633:bool)
        n78 = Negate(x=w935) -> (-x=w933:dbl)
        n79 = Or(x=w633, y="Mode4_manual\n(get now ang)") -> (x .or. y?=w631:bool)
        n80 = case shown="참" w631 {
          frame False {
          }
          frame True {
            w1461 = 0.0 ("angle")
            n81 = local write "AngNowCmd"(w1461) -> ()
            n82 = local write "fine_tunning"(w1461) -> ()
            n83 = local write "delta_ang_memo"(w1461) -> ()
            n84 = local write "angle"(w1461) -> ()
            n85 = local write "Target_V"(w1461) -> ()
            n86 = local write "nowphi"(w1461) -> ()
          }
        }
        n87 = feedback #1(w946) -> (w945:dbl)
        n88 = feedback #2(w946) -> (w944:dbl)
        n89 = local read "delta_ang_memo"() -> (w938:dbl)
        n90 = feedback #3(w946) -> (w943:dbl)
        n91 = Compound Arithmetic op=ADD(w945, w944, w943) -> (w942:dbl)
        n92 = Divide(x=w942, y=3.0) -> (x/y=w867:dbl)
        n93 = local read "nowphi"() -> (w870:dbl)
        n94 = local read "DriveMODE"() -> (w402:dbl)
        n95 = local read "SteerAng"() -> (w375:dbl)
        n96 = Tick Count (ms)() -> (millisecond timer value=w924:u32)
        "time_now" <- w924
        n97 = feedback #4(0.0 ("phi_d")) -> (w922:dbl)
        "delta_ang_memo" <- w922
        n98 = Add(x=w639, y=w922) -> (x+y=w909:dbl)
        n99 = formula code="if (u >165)\ny=165;\nelse if (u <-165)\ny=-165;\nelse\ny=u;"("u"=w909) -> ("y"=w866:dbl)
        n100 = local read "Time_int"() -> (w1021:i32)
        n101 = Equal?(x=w402, y=4.0) -> (x = y?=w351:bool)
        n102 = feedback #5() -> (w1063:u32)  [unwired: 1 in]
        n103 = feedback-in #5(w924) -> ()
        n104 = Subtract(x=w924, y=w1063) -> ()  [unwired: 1 out]
        n105 = local read "driveONoFF"() -> (w960:dbl)
        n106 = local read "fine_tunning"() -> (w956:sgl)
        n107 = Add(x=w870, y="nowphi_in") -> (x+y=w868:dbl)
        n108 = formula code="phi_d=phi_t-phi_n;\nif (abs(phi_d) < 0.05)\nphi_d=0;\nelse \nphi_d=phi_d;"("phi_n"=w868, "phi_t"="phi_target") -> ("phi_d"=w952:dbl)
        n109 = Divide(x=w1021, y=u32 1000) -> (x/y=w377:dbl)
        n110 = Add(x=w933, y=0.0) -> (x+y=w939:dbl)
        n111 = Equal?(x=w956, y=1.0) -> (x = y?=w958:bool)
        n112 = formula code="if ( 180 < u && y <=360)\ny = u-360;\nelse\ny = u;"("u"=w939) -> ("y"=w482:dbl)
        "AngNowFB" <- w482
        n113 = Equal?(x=w960, y=1.0) -> (x = y?=w620:bool)
        n114 = local read "Target_V"() -> (w638:dbl)
        n115 = formula code="float phi_cmd,phi;\nphi=now_phi+ref_phi;\nif ( 180 < phi && phi <=360)\nphi_cmd = phi-360;\nelse\nphi_cmd = phi;"("ref_phi"=w866, "now_phi"=w867) -> ("phi_cmd"=w926:dbl)
        n116 = local read "AutoSBCOn"() -> (w618:bool)
        n117 = Select(t=w620, s=w618, f="DriveStart_manual") -> (s? t:f=w613:bool)
        n118 = feedback #6(0.0) -> (w617:dbl)
        n119 = case shown="거짓" w613 {
          tunnel: w377 -> [w1167 _]
          tunnel: [w1167 w1168] -> w616
          tunnel: w617 -> [_ w1168]
          frame False {
          }
          frame True {
          }
        }
        n120 = feedback-in #6(w616) -> ()
        n121 = Subtract(x=w377, y=w616) -> (x-y=w354:dbl)
        n122 = Greater?(x=w354, y=w347) -> (0:w614:bool)
        n123 = And(x=w614, y=w613) -> (x .and. y?=w502:bool)
        n124 = feedback #7(0.0) -> (w971:dbl)
        n125 = case shown="참" w958 {
          tunnel: w377 -> [w1486 _]
          tunnel: [w1486 w1487] -> w972
          tunnel: w971 -> [_ w1487]
          frame False {
          }
          frame True {
          }
        }
        n126 = feedback-in #7(w972) -> ()
        n127 = Subtract(x=w377, y=w972) -> (x-y=w951:dbl)
        n128 = Greater?(x=w951, y=0.0) -> (0:w968:bool)
        n129 = Less?(x=w951, y=0.1) -> (x < y?=w967:bool)
        n130 = And(x=w968, y=w967) -> (x .and. y?=w940:bool)
        n131 = case shown="참" w940 {
          tunnel: w952 -> [_ w1485]
          tunnel: [w1484 w1485] -> w962
          tunnel: w938 -> [w1484 _]
          frame False {
          }
          frame True {
          }
        }
        n132 = feedback-in #4(w962) -> ()
        n133 = Select(t=w638, s=w618, f="V*manualn") -> (s? t:f=w484:dbl)
        n134 = local read "DriveMODE"() -> (w835:dbl)
        n135 = feedback #8(0.0) -> (w399:dbl)
        n136 = Equal?(x=w835, y=3.0) -> (x = y?=w834:bool)
        n137 = Greater?(x=w354, y=0.5) -> (0:w355:bool)
        n138 = Greater?(x=w354, y=w604) -> (0:w603:bool)
        n139 = Less?(x=w354, y=w347) -> (x < y?=w356:bool)
        n140 = Less?(x=w354, y=w347) -> (x < y?=w602:bool)
        n141 = Greater?(x=w354, y=0.0) -> (0:w361:bool)
        n142 = Greater?(x=w354, y=w408) -> (0:w612:bool)
        n143 = Less?(x=w354, y=w347) -> (x < y?=w360:bool)
        n144 = Less?(x=w354, y=w347) -> (x < y?=w611:bool)
        n145 = Greater?(x=w354, y=1.5) -> (0:w499:bool)
        n146 = Less?(x=w354, y=w604) -> (x < y?=w605:bool)
        n147 = Greater?(x=w951, y=0.0) -> (0:w965:bool)
        n148 = And(x=w603, y=w602) -> (x .and. y?=w601:bool)
        n149 = And(x=w612, y=w611) -> (x .and. y?=w352:bool)
        n150 = And(x=w355, y=w356) -> (x .and. y?=w345:bool)
        n151 = Compound Arithmetic op=AND ("복합 연산")(w499, w605) -> (w344:bool)
        n152 = Select(t=w484, s=w834, f=-1.0 ("input variable")) -> ()  [unwired: 1 out]
        n153 = And(x=w361, y=w360) -> (x .and. y?=w346:bool)
        n154 = Less?(x=w951, y=0.003) -> (x < y?=w966:bool)
        n155 = Greater?(x=w354, y=0.2) -> (0:w498:bool)
        n156 = Less?(x=w354, y=w408) -> (x < y?=w497:bool)
        n157 = Add(x="ang_compensate", y=w926) -> (x+y=w910:dbl)
        n158 = call <vilib>:"Write Read.vi"("Byte Count"=u32 6, "error in (no error)"=w1003, "Bytes to Write"=u8[] [168], "Slave Address (7-bit)"=w1002, "I2C Ref In"=w1004) -> ("error out"=w1001:errorcluster, "Bytes Read"=w1019:u8[])  [unwired: 3 in, 1 out]
        n159 = And(x=w965, y=w966) -> (x .and. y?=w851:bool)
        n160 = Or(x=w631, y=w851) -> (x .or. y?=w950:bool)
        n161 = case shown="거짓" w950 {
          tunnel: [w1464 w1465] -> w948
          tunnel: w944 -> [w1464 _]
          tunnel: w933 -> [_ w1465]
          frame False {
          }
          frame True {
          }
        }
        n162 = case shown="거짓" w950 {
          tunnel: w933 -> [_ w1467]
          tunnel: [w1466 w1467] -> w949
          tunnel: w943 -> [w1466 _]
          frame False {
          }
          frame True {
          }
        }
        n163 = case shown="거짓" w950 {
          tunnel: w933 -> [_ w1463]
          tunnel: [w1462 w1463] -> w947
          tunnel: w945 -> [w1462 _]
          frame False {
          }
          frame True {
          }
        }
        n164 = feedback-in #1(w947) -> ()
        n165 = feedback-in #2(w948) -> ()
        n166 = feedback-in #3(w949) -> ()
        n167 = And(x=w498, y=w497) -> (x .and. y?=w500:bool)
        n168 = feedback #9(0.0) -> (w842:dbl)
        n169 = Index Array "Index Array"(array=w1019) -> (element #1=w1014:u8, element #2=w1013:u8, element #3=w1012:u8, element #4=w1011:u8, element #5=w1010:u8, element #6=w1009:u8)  [unwired: 6 in]
        n170 = Or(x=w851, y=w631) -> (x .or. y?=w711:bool)
        n171 = feedback #10(0.0) -> (w850:dbl)
        n172 = feedback #11(0.0) -> (w917:dbl)
        n173 = feedback-in #11(w910) -> ()
        n174 = feedback #12(0.0) -> (w495:dbl)
        n175 = Join Numbers(hi=w1013, lo=w1014) -> ((hi.lo)=w1017:u16)
        n176 = Join Numbers(hi=w1011, lo=w1012) -> ((hi.lo)=w1016:u16)
        n177 = Join Numbers(hi=w1009, lo=w1010) -> ((hi.lo)=w1015:u16)
        n178 = feedback #13(0.0) -> (w985:dbl)
        n179 = feedback #14(0.0) -> (w391:dbl)
        n180 = To Word Integer(number=w1017) -> ()  [unwired: 1 out]
        n181 = To Word Integer(number=w1016) -> ()  [unwired: 1 out]
        n182 = To Word Integer(number=w1015) -> (16bit integer=w1018:i16)
        "Z rate" <- w1018
        n183 = local read "l_rear"() -> (w324:dbl)
        "dist_avr" <- w324
        n184 = Greater?(x=w324, y=5.0) -> (0:w864:bool)
        n185 = Multiply(x="ref_LFP_cut", y=6.283185307179586) -> (x*y=w916:dbl)
        n186 = Greater?(x=w377, y=42.0) -> (0:w338:bool)
        n187 = And(x=w351, y=w338) -> (x .and. y?=w353:bool)
        n188 = case shown="거짓" w353 {
          tunnel: w399 -> [w1159 _]
          tunnel: [w1159 w1160] -> w400
          tunnel: w377 -> [_ w1160]
          frame False {
          }
          frame True {
          }
        }
        n189 = feedback-in #8(w400) -> ()
        n190 = Subtract(x=w377, y=w400) -> (x-y=w339:dbl)
        n191 = Greater?(x=w339, y=3.0) -> (0:w394:bool)
        n192 = Less?(x=w339, y=3.03) -> (x < y?=w395:bool)
        n193 = And(x=w394, y=w395) -> (x .and. y?=w393:bool)
        n194 = case shown="거짓" w393 {
          tunnel: w391 -> [w1157 _]
          tunnel: [w1157 w1158] -> w370
          tunnel: w375 -> [_ w1158]
          frame False {
          }
          frame True {
          }
        }
        n195 = feedback-in #14(w370) -> ()
        n196 = Multiply(x="PD_cut_rot 2", y=6.283185307179586) -> (x*y=w982:dbl)
        n197 = Reciprocal(x=w916) -> (1/x=w914:dbl)
        n198 = Subtract(x="SteerOri", y=w370) -> (x-y=w385:dbl)
        n199 = Reciprocal(x=w982) -> (1/x=w983:dbl)
        n200 = Divide(x=w1018, y=65535.0 ("gyroscale")) -> (x/y=w1005:dbl)
        n201 = Greater?(x=w339, y=3.0) -> (0:w389:bool)
        n202 = Less?(x=w339, y=6.0) -> (x < y?=w388:bool)
        n203 = Compound Arithmetic op=AND ("복합 연산")(w389, w388, w338) -> (w378:bool)
        n204 = Or(x=w378, y=w352) -> (x .or. y?=w383:bool)
        n205 = feedback #15(0.0) -> (w989:dbl)
        n206 = Divide(x=w385, y="deg/Volt") -> (x/y=w382:dbl)
        n207 = local read "DriveMODE"() -> (w434:dbl)
        "DriveMode" <- w434
        n208 = Equal?(x=w434, y=5.0) -> (x = y?=w862:bool)
        n209 = And(x=w864, y=w862) -> (x .and. y?=w860:bool)
        n210 = case shown="거짓" w860 {
          tunnel: w377 -> [w1443 _]
          tunnel: [w1443 w1444] -> w849
          tunnel: w850 -> [_ w1444]
          frame False {
          }
          frame True {
          }
        }
        n211 = feedback-in #10(w849) -> ()
        n212 = Subtract(x=w377, y=w849) -> (x-y=w844:dbl)
        n213 = Less?(x=w844, y=0.01) -> (x < y?=w848:bool)
        n214 = Greater?(x=w844, y=0.0) -> (0:w847:bool)
        n215 = And(x=w847, y=w848) -> (x .and. y?=w840:bool)
        n216 = case shown="거짓" w840 {
          tunnel: w377 -> [_ w1440]
          tunnel: [w1439 w1440] -> w843
          tunnel: w842 -> [w1439 _]
          frame False {
          }
          frame True {
          }
        }
        n217 = feedback-in #9(w843) -> ()
        n218 = Subtract(x=w377, y=w843) -> (x-y=w839:dbl)
        "Back driving time" <- w839
        n219 = Greater?(x=w839, y=0.0) -> (0:w857:bool)
        n220 = Less?(x=w839, y=25.0) -> (x < y?=w856:bool)
        n221 = And(x=w857, y=w856) -> (x .and. y?=w838:bool)
        "back driving act" <- w838
        n222 = formula code="if (u >= lim*1)\ny0=lim*1;\nelse if (u <= -lim*1)\ny0=-lim*1;\nelse\ny0=u;"("u"=w382, "lim"=2.0 ("입력 변수")) -> ("y0"=w368:dbl)
        "IniSteerCmd" <- w368
        n223 = feedback #16(0.0) -> (w918:dbl)
        n224 = formula code="float F,A,B,C,y0;\nF=2*tau+T;\nA=(2*a+b*T)/F;\nB=(b*T-2*a)/F;\nC=(2*tau-T)/F;\ny0=A*u0+B*u1+C*y1;"("tau"=w914, "u0"=w910, "u1"=w917, "y1"=w918, "T"=0.001 ("input variable"), "a"=0.0 ("input variable"), "b"=1.0 ("input variable")) -> ("y0"=w483:dbl)
        "AngNowCmd" <- w483
        n225 = Subtract(x=w483, y=w482) -> (x-y=w323:dbl)
        "PhiErr" <- w323
        n226 = formula code="if (phi_err > 3)\nerr=3;\nelse if (phi_err < -3)\nerr=-3;\nelse\nerr=phi_err;"("phi_err"=w323) -> ("err"=w975:dbl)
        n227 = Bundle(w483, "y"=w482, w323) -> (→"Ang":cluster{dbl, "y":dbl, dbl})  [unwired: 1 in]
        n228 = case shown="참" w500 {
          tunnel: w323 -> [_ w1164]
          tunnel: [w1163 w1164] -> w350
          tunnel: w495 -> [w1163 _]
          frame False {
          }
          frame True {
          }
        }
        "AngError" <- w350
        n229 = feedback-in #12(w350) -> ()
        n230 = feedback-in #13(w975) -> ()
        n231 = formula code="float F,A,B,C,ykd,ykp,y0;\nF=2*tau+T;\nA=(2*Kd_rot)/F;\nB=(-2*Kd_rot)/F;\nC=(2*tau-T)/F;\nykd=A*u0+B*u1+C*y1;\nykp=Kp_rot*u0;\ny0=ykp+ykd;"("tau"=w983, "u0"=w975, "u1"=w985, "y1"=w989, "T"=0.001 ("input variable"), "Kp_rot"="Kp_rot 3", "Kd_rot"="Kd_rot 4") -> ("y0"=w992:dbl)
        n232 = formula code="if (phi_ref > cri_ang1 && phi_ref < cri_ang2)\nini_phi = steer1;\nelse if (phi_ref > cri_ang2)\nini_phi = steer2;\nelse if (phi_ref < -cri_ang1 && phi_ref > -cri_ang2)\nini_phi = -steer1;\nelse if (phi_ref < -cri_ang2)\nini_phi =  -steer2;\nelse \nini_phi = 0;"("phi_ref"=w350, "steer1"="ini_phi_1", "steer2"="ini_phi_2", "cri_ang1"="criteria ang1", "cri_ang2"="criteria ang2") -> ("ini_phi"=w367:dbl)
        n233 = feedback-in #15(w992) -> ()
        n234 = Add(x=0.0, y=w992) -> (x+y=w979:dbl)
        "YRRef" <- w979
        n235 = feedback-in #16(w483) -> ()
        n236 = Negate(x="KpStopError") -> (-x=w404:dbl)
        n237 = Greater?(x=w339, y=3.1) -> (0:w372:bool)
        n238 = Less?(x=w339, y=5.8) -> (x < y?=w371:bool)
        n239 = Greater Than 0?(x=w350) -> (x > 0?=w406:bool)
        n240 = Compound Arithmetic op=AND ("복합 연산")(w372, w371, w338) -> (w337:bool)
        n241 = Select(t="KpStopError", s=w406, f=w404) -> (s? t:f=w407:dbl)
        n242 = Greater?(x=w324, y="Desire back dist") -> (0:w853:bool)
        n243 = And(x=w853, y=w838) -> (x .and. y?=w510:bool)
        "back stop" <- w510
        n244 = feedback #17(0.0) -> (w545:dbl)
        n245 = case shown="거짓" w510 {
          tunnel: w545 -> [_ w1166]
          tunnel: [w1165 w1166] -> w543
          tunnel: w377 -> [w1165 _]
          frame False {
          }
          frame True {
          }
        }
        n246 = feedback-in #17(w543) -> ()
        n247 = Multiply(x=w407, y=w323) -> (x*y=w403:dbl)
        n248 = Subtract(x=w377, y=w543) -> (x-y=w542:dbl)
        n249 = formula code="float V_now;\nV_now=acc_d*t;\n\nif (V_now <= V_targ )\nV_in=V_targ;\nelse \nV_in = V_now;"("V_targ"=-1.2 ("입력 변수"), "acc_d"=-0.3 ("입력 변수"), "t"=w542) -> ("V_in"=w532:dbl)
        n250 = Or(x=w345, y=w337) -> (x .or. y?=w358:bool)
        n251 = Select(t=w367, s=w344, f=w366) -> (s? t:f=w365:dbl)
        n252 = Multiply(x="PD_cut_rot", y=6.283185307179586) -> (x*y=w1085:dbl)
        n253 = feedback #18(0.0) -> (w1082:dbl)
        n254 = Reciprocal(x=w1085) -> (1/x=w1084:dbl)
        n255 = local read "Kt_rot"() -> (w929:dbl)
        n256 = Multiply(x="FF_cut", y=6.283185307179586) -> (x*y=w1106:dbl)
        n257 = Equal?(x=w434, y=w832) -> (x = y?=w831:bool)
        n258 = Select(t=w366, s=w601, f=w365) -> (s? t:f=w369:dbl)
        n259 = feedback #19(0.0 ("gy_z[]")) -> (w1095:dbl)
        n260 = formula code="if (u >= lim*1)\ny0=lim*1;\nelse if (u <= -lim*1)\ny0=-lim*1;\nelse\ny0=u;"("u"=w403, "lim"="LimStopErrVel") -> ("y0"=w437:dbl)
        n261 = Reciprocal(x=w1106) -> (1/x=w1104:dbl)
        n262 = Greater?(x=w339, y=3.2) -> (0:w342:bool)
        n263 = Less?(x=w339, y=5.9) -> (x < y?=w343:bool)
        n264 = Or(x=w831, y=w510) -> ()  [unwired: 1 out]
        n265 = Compound Arithmetic op=AND ("복합 연산")(w342, w343, w338) -> (w336:bool)
        n266 = Not Equal?(x=w434, y=w832) -> (x != y?=w833:bool)
        n267 = Divide(x="Jm_rotFF", y=w929) -> (x/y=w1062:dbl)
        n268 = And(x=w833, y=w510) -> (x .and. y?=w380:bool)
        n269 = Select(t=w368, s=w336, f=w369) -> (s? t:f=w379:dbl)
        n270 = Divide(x="Bm_rot FF", y=w929) -> (x/y=w1061:dbl)
        n271 = case shown="참" w380 {
          tunnel: [FALSE TRUE] -> w348
          frame False {
          }
          frame True {
          }
        }
        n272 = case shown="2" w434 {
          tunnel: [TRUE TRUE TRUE FALSE] -> w349
          tunnel: [TRUE FALSE TRUE FALSE] -> w855
          tunnel: [TRUE FALSE TRUE FALSE] -> _
          tunnel: [TRUE FALSE TRUE FALSE] -> w854
          frame 1 {
          }
          frame 2 {
          }
          frame 3 {
          }
          frame 5, Default {
          }
        }
        n273 = Multiply(x="Cut_StopErr", y=6.283185307179586) -> (x*y=w599:dbl)
        n274 = feedback #20(0.0 ("Vel_cmd\n(False) 2")) -> (w595:dbl)
        n275 = feedback-in #20(w437) -> ()
        n276 = Or(x="Enc_set 0", y=w711) -> (x .or. y?=w712:bool)
        n277 = Multiply(x="StRefCut", y=6.283185307179586) -> (x*y=w582:dbl)
        n278 = local read "YawConton"() -> (w955:bool)
        n279 = Reciprocal(x=w599) -> (1/x=w597:dbl)
        n280 = feedback #21(0.0 ("gy_z[]")) -> (w1103:dbl)
        n281 = feedback #22(0.0 ("Vel_cmd\n(False) 2")) -> (w578:dbl)
        n282 = feedback-in #22(w379) -> ()
        n283 = Reciprocal(x=w582) -> (1/x=w580:dbl)
        n284 = feedback #23(0.0) -> (w1077:dbl)
        n285 = Multiply(x=w484, y="ShiftVelcrit") -> (x*y=w491:dbl)
        n286 = Or(x=w854, y=w348) -> (x .or. y?=w363:bool)
        n287 = Or(x=w855, y=w348) -> ()  [unwired: 1 out]
        n288 = xnode "Left encoder 4"("Reset Counter"=w712) -> ("Counter Value"=w775:i32)  [unwired: 1 in, 3 out]
        n289 = xnode "Encoder 2"("Reset Counter"=w712) -> ("Counter Value"=w774:i32)  [unwired: 1 in, 3 out]
        n290 = xnode "Left encoder 2"("Reset Counter"=w712) -> ("Counter Value"=w770:i32)  [unwired: 1 in, 3 out]
        n291 = xnode "Left encoder 3"("Reset Counter"="Enc_steer") -> ("Counter Value"=w755:i32)  [unwired: 1 in, 3 out]
        n292 = feedback #24(0.0) -> (w579:dbl)
        n293 = formula code="float F,A,B,C,y0;\nF=2*tau+T;\nA=(2*a+b*T)/F;\nB=(b*T-2*a)/F;\nC=(2*tau-T)/F;\ny0=A*u0+B*u1+C*y1;"("tau"=w580, "u0"=w379, "u1"=w578, "y1"=w579, "T"=0.001 ("입력 변수"), "a"=0.0 ("입력 변수"), "b"=1.0 ("입력 변수")) -> ("y0"=w438:dbl)
        n294 = feedback-in #24(w438) -> ()
        n295 = Select(t=w484, s=w502, f=0.0) -> (s? t:f=w487:dbl)
        "Vref" <- w487
        n296 = local write "From_SBC_DOB"(w363) -> ()
        n297 = feedback #25(0.0) -> (w596:dbl)
        n298 = formula code="float F,A,B,C,y0;\nF=2*tau+T;\nA=(2*a+b*T)/F;\nB=(b*T-2*a)/F;\nC=(2*tau-T)/F;\ny0=A*u0+B*u1+C*y1;"("tau"=w597, "u0"=w437, "u1"=w595, "y1"=w596, "T"=0.001 ("입력 변수"), "a"=0.0 ("입력 변수"), "b"=1.0 ("입력 변수")) -> ("y0"=w525:dbl)
        n299 = feedback-in #25(w525) -> ()
        n300 = Multiply(x=w774, y=6.283185307179586) -> (x*y=w803:dbl)
        n301 = Divide(x=w803, y=40000.0) -> (x/y=w442:dbl)
        n302 = Negate(x=w775) -> (-x=w776:i32)
        n303 = Multiply(x=w770, y=6.283185307179586) -> (x*y=w772:dbl)
        n304 = Multiply(x=w776, y=6.283185307179586) -> (x*y=w800:dbl)
        n305 = Multiply(x=w755, y=6.283185307179586) -> (x*y=w759:dbl)
        n306 = Absolute Value(x=w491) -> (abs(x)=w490:dbl)
        n307 = local read "Vel_Robot"() -> (w650:dbl)
        n308 = Divide(x=w772, y=40000.0) -> (x/y=w715:dbl)
        n309 = Divide(x=w800, y=40000.0) -> (x/y=w441:dbl)
        n310 = Divide(x=w759, y=524288.0) -> (x/y=w756:dbl)
        n311 = Divide(x=w756, y=-100.0) -> (x/y=→"th_steer":dbl)
        n312 = feedback #26(0.0 ("gy_ratelimit")) -> (w730:dbl)
        n313 = feedback #27(0.0 ("gy_ratelimit")) -> (w753:dbl)
        n314 = feedback #28(0.0 ("gy_ratelimit")) -> (w731:dbl)
        n315 = Greater?(x=w650, y=0.0) -> (0:w652:bool)
        n316 = Not(x=w346) -> (.not. x?=w364:bool)
        n317 = feedback #29(0.0) -> (w728:dbl)
        n318 = feedback #30(0.0) -> (w748:dbl)
        n319 = feedback #31(0.0) -> (w733:dbl)
        n320 = feedback #32(0.0) -> (w519:dbl)
        n321 = Multiply(x="Wheelvel_ratelimit cut", y=6.283185307179586) -> (x*y=w750:dbl)
        n322 = local read "Vel_Robot"() -> (w623:dbl)
        n323 = And(x=w364, y=w363) -> (x .and. y?=w362:bool)
        n324 = Bundle(w442, w441, w715) -> (w783:cluster{dbl, dbl, dbl})  [unwired: 1 in]
        n325 = Reciprocal(x=w750) -> (1/x=w720:dbl)
        n326 = feedback #33(0.0) -> (w691:dbl)
        n327 = Or(x="Drive_Enable", y=w349) -> (x .or. y?=w511:bool)
        n328 = Or(x=w511, y="Rear_DriveE") -> (x .or. y?=w332:bool)
        n329 = Absolute Value(x=w623) -> (abs(x)=w622:dbl)
        n330 = Greater?(x=w622, y=0.02) -> (0:w621:bool)
        n331 = Select(t="YR*_Off(manual)", s=w621, f=FALSE) -> (s? t:f=w625:bool)
        n332 = Select(t=w979, s=w625, f=0.0) -> (s? t:f=w978:dbl)
        "YRRefOn" <- w978
        n333 = feedback-in #19(w978) -> ()
        n334 = formula code="float F,A,B,C,y0;\nF=2*tau+T;\nA=(2*a+b*T)/F;\nB=(b*T-2*a)/F;\nC=(2*tau-T)/F;\ny0=A*u0+B*u1+C*y1;"("tau"=w1104, "u0"=w978, "u1"=w1095, "y1"=w1103, "T"=0.001 ("input variable"), "a"=w1062, "b"=w1061) -> ("y0"=w1076:dbl)
        "RotFF" <- w1076
        n335 = feedback-in #21(w1076) -> ()
        n336 = Not(x=w380) -> (.not. x?=w569:bool)
        n337 = Not(x=w344) -> (.not. x?=w572:bool)
        n338 = Compound Arithmetic op=OR ("복합 연산")("Rear_steerEnable", w362, w358) -> (w331:bool)
        "StEn" <- w331
        n339 = Divide(x=w783, y=6.0) -> (x/y=w781:cluster{dbl, dbl, dbl})
        n340 = local read "Abs angle or gyro"() -> (w411:dbl)
        "ori_phi" <- w411
        n341 = Multiply(x=w781, y=0.125) -> (x*y=w780:cluster{dbl, dbl, dbl})
        n342 = Compound Arithmetic op=OR ("복합 연산")(w511, "Front enable", w348) -> (w535:bool)
        n343 = Not(x=w383) -> (.not. x?=w534:bool)
        n344 = Unbundle(w780) -> (→"l_R 2":dbl, →"l_L 2":dbl, →"l_rear":dbl)
        n345 = And(x=w534, y=w535) -> (x .and. y?=w334:bool)
        "DEn" <- w334
        n346 = local read "Readyon"() -> (w325:bool)
        n347 = feedback #34(0.0) -> (w794:dbl)
        n348 = feedback-in #34(w442) -> ()
        n349 = feedback #35(0.0) -> (w788:dbl)
        n350 = feedback-in #35(w441) -> ()
        n351 = feedback #36(0.0) -> (w762:dbl)
        n352 = feedback-in #36(w715) -> ()
        n353 = feedback #37(0.0) -> (w729:dbl)
        n354 = feedback #38(0.0) -> (w752:dbl)
        n355 = feedback #39(0.0) -> (w732:dbl)
        n356 = Boolean To (0,1)(Boolean=w332) -> (0, 1=w333:i16)
        n357 = formula code="if (ang > 360)\nang1=ang-360;\nelse\nang1=ang;"("ang"=w411) -> ("ang1"=w413:dbl)
        n358 = formula code="float phi;\nif (sensor > 180 && sensor <= 360)\nphi = sensor-360;\nelse\nphi = sensor;"("sensor"=w413) -> ("phi"=w412:dbl)
        n359 = xnode "Digital output (1 sample) 3"("C/DIO5 (DIO5)"=w334, "A/DIO2 (Pin 15)"=w331, "C/DIO7 (DIO7)"=w325) -> ()  [unwired: 1 in, 1 out]
        n360 = Multiply(x=i16 5, y=w333) -> (x*y=w330:i16)
        "RearEn" <- w330
        n361 = feedback #40(0.0) -> (w1111:dbl)
        n362 = feedback #41(0.0 ("gy_z[]")) -> (w1108:dbl)
        n363 = Multiply(x="Vel_cut", y=6.283185307179586) -> (x*y=w766:dbl)
        n364 = Multiply(x="Vel_cut", y=6.283185307179586) -> (x*y=w792:dbl)
        n365 = xnode "Analog output (1 sample) 3"("B/AO1 (Pin 4)"=w330) -> ()  [unwired: 1 in, 1 out]
        n366 = Multiply(x="Vel_cut", y=6.283185307179586) -> (x*y=w797:dbl)
        n367 = Reciprocal(x=w766) -> (1/x=w768:dbl)
        n368 = Reciprocal(x=w792) -> (1/x=w790:dbl)
        n369 = Reciprocal(x=w797) -> (1/x=w796:dbl)
        n370 = feedback #42(0.0 ("gy_ratelimit")) -> (w1040:dbl)
        n371 = Select(t="sigma_rate", s=w502, f=w682) -> (s? t:f=w685:dbl)
        n372 = Divide(x="Jm_rot", y="Kt_rot") -> (x/y=w1102:dbl)
        n373 = Multiply(x="DOB_FB_cut", y=6.283185307179586) -> (x*y=w1112:dbl)
        n374 = feedback #43(0.0) -> (w683:dbl)
        n375 = Select(t=w683, s=w502, f=w682) -> (s? t:f=w684:dbl)
        n376 = Add(x=w685, y=w684) -> (x+y=w679:dbl)
        "Sigmafor V+ySigma=Vw" <- w679
        n377 = Reciprocal(x=w1112) -> (1/x=w1114:dbl)
        n378 = Less?(x=w679, y="Vw*limitby_sigma") -> (x < y?=w693:bool)
        n379 = feedback #44(0.0) -> (w1033:dbl)
        n380 = Divide(x="Bm_rot", y="Kt_rot") -> (x/y=w1101:dbl)
        n381 = Select(t=w679, s=w693, f="Vw*limitby_sigma") -> (s? t:f=w694:dbl)
        n382 = feedback-in #43(w694) -> ()
        n383 = Greater?(x=w700, y=30000) -> (0:w997:bool)
        n384 = feedback #45(w763) -> (w769:dbl)
        n385 = formula code="y0=(2*(u0-u1)-(T-2*Tau)*y1)/(T+2*Tau);"("Tau"=w768, "u0"=w715, "u1"=w762, "y1"=w769, "T"=w765) -> ("y0"=w718:dbl)
        n386 = feedback-in #45(w718) -> ()
        n387 = feedback #46(w763) -> (w789:dbl)
        n388 = formula code="y0=(2*(u0-u1)-(T-2*Tau)*y1)/(T+2*Tau);"("Tau"=w790, "u0"=w441, "u1"=w788, "y1"=w789, "T"=w765) -> ("y0"=w786:dbl)
        n389 = feedback-in #46(w786) -> ()
        n390 = Greater?(x=w700, y=180000) -> (0:w897:bool)
        n391 = Greater?(x=w700, y=50000) -> (0:w907:bool)
        n392 = Greater?(x=w700, y=150000) -> (0:w900:bool)
        n393 = Greater?(x=w700, y=40000) -> (0:w999:bool)
        n394 = Greater?(x=w700, y=60000) -> (0:w904:bool)
        n395 = Multiply(x="ratelimit cut", y=6.283185307179586) -> (x*y=w1036:dbl)
        n396 = feedback #47(w763) -> (w795:dbl)
        n397 = formula code="y0=(2*(u0-u1)-(T-2*Tau)*y1)/(T+2*Tau);"("Tau"=w796, "u0"=w442, "u1"=w794, "y1"=w795, "T"=w765) -> ("y0"=w782:dbl)
        n398 = feedback-in #47(w782) -> ()
        n399 = Reciprocal(x=w1036) -> (1/x=w1035:dbl)
        n400 = feedback #48(0.0) -> (w1110:dbl)
        n401 = feedback #49(0.0) -> (w1107:dbl)
        n402 = Bundle("y0"=w782, "y0"=w786, "y0"=w718) -> (w777:cluster{"y0":dbl, "y0":dbl, "y0":dbl})  [unwired: 1 in]
        n403 = feedback #50(w878) -> (w896:dbl)
        n404 = case shown="참" w897 {
          tunnel: w412 -> [w1453 _]
          tunnel: [w1453 w1454] -> w895
          tunnel: w896 -> [_ w1454]
          frame False {
          }
          frame True {
          }
        }
        n405 = feedback-in #50(w895) -> ()
        n406 = feedback #51(w878) -> (w908:dbl)
        n407 = case shown="참" w907 {
          tunnel: w412 -> [w1459 _]
          tunnel: [w1459 w1460] -> w327
          tunnel: w908 -> [_ w1460]
          frame False {
          }
          frame True {
          }
        }
        n408 = feedback-in #51(w327) -> ()
        n409 = feedback #52(w878) -> (w901:dbl)
        n410 = case shown="참" w900 {
          tunnel: w412 -> [w1455 _]
          tunnel: [w1455 w1456] -> w902
          tunnel: w901 -> [_ w1456]
          frame False {
          }
          frame True {
          }
        }
        n411 = feedback-in #52(w902) -> ()
        n412 = feedback #53(w878) -> (w996:dbl)
        n413 = case shown="참" w999 {
          tunnel: w412 -> [w1498 _]
          tunnel: [w1498 w1499] -> w876
          tunnel: w996 -> [_ w1499]
          frame False {
          }
          frame True {
          }
        }
        n414 = feedback-in #53(w876) -> ()
        n415 = feedback #54(w878) -> (w903:dbl)
        n416 = case shown="참" w904 {
          tunnel: w412 -> [w1457 _]
          tunnel: [w1457 w1458] -> w328
          tunnel: w903 -> [_ w1458]
          frame False {
          }
          frame True {
          }
        }
        n417 = feedback-in #54(w328) -> ()
        n418 = feedback #55(0.0) -> (w1038:dbl)
        n419 = Divide(x=w777, y=6.0) -> (x/y=w445:cluster{"y0":dbl, "y0":dbl, "y0":dbl})
        n420 = Multiply(x=w445, y=0.125) -> (x*y=w714:cluster{"y0":dbl, "y0":dbl, "y0":dbl})
        n421 = Unbundle(w714) -> ("y0"=w452:dbl, "y0"=w454:dbl, "y0"=w453:dbl)
        n422 = formula code="float rate;\nrate=gy-gy_r1;\nif (rate > limit)\ngy_ratelimit=gy_r1+limit;\nelse if (rate < -limit)\ngy_ratelimit=gy_r1+(-limit);\nelse\ngy_ratelimit=gy;"("gy"=w453, "gy_r1"=w730, "limit"="wheelV_ratelimit") -> ("gy_ratelimit"=w721:dbl)
        n423 = formula code="float rate;\nrate=gy-gy_r1;\nif (rate > limit)\ngy_ratelimit=gy_r1+limit;\nelse if (rate < -limit)\ngy_ratelimit=gy_r1+(-limit);\nelse\ngy_ratelimit=gy;"("gy"=w452, "gy_r1"=w753, "limit"="wheelV_ratelimit") -> ("gy_ratelimit"=w741:dbl)
        n424 = formula code="float rate;\nrate=gy-gy_r1;\nif (rate > limit)\ngy_ratelimit=gy_r1+limit;\nelse if (rate < -limit)\ngy_ratelimit=gy_r1+(-limit);\nelse\ngy_ratelimit=gy;"("gy"=w454, "gy_r1"=w731, "limit"="wheelV_ratelimit") -> ("gy_ratelimit"=w740:dbl)
        n425 = feedback-in #26(w721) -> ()
        n426 = feedback-in #27(w741) -> ()
        n427 = feedback-in #28(w740) -> ()
        n428 = feedback-in #29(w721) -> ()
        n429 = feedback-in #30(w741) -> ()
        n430 = feedback-in #31(w740) -> ()
        n431 = formula code="float F,A,B,C,y0;\nF=2*tau+T;\nA=(2*a+b*T)/F;\nB=(b*T-2*a)/F;\nC=(2*tau-T)/F;\ny0=A*u0+B*u1+C*y1;"("tau"=w720, "u0"=w721, "u1"=w728, "y1"=w729, "T"=0.001 ("input variable"), "a"=0.0 ("input variable"), "b"=1.0 ("input variable")) -> ("y0"=w449:dbl)
        n432 = formula code="float F,A,B,C,y0;\nF=2*tau+T;\nA=(2*a+b*T)/F;\nB=(b*T-2*a)/F;\nC=(2*tau-T)/F;\ny0=A*u0+B*u1+C*y1;"("tau"=w720, "u0"=w741, "u1"=w748, "y1"=w752, "T"=0.001 ("input variable"), "a"=0.0 ("input variable"), "b"=1.0 ("input variable")) -> ("y0"=w451:dbl)
        n433 = formula code="float F,A,B,C,y0;\nF=2*tau+T;\nA=(2*a+b*T)/F;\nB=(b*T-2*a)/F;\nC=(2*tau-T)/F;\ny0=A*u0+B*u1+C*y1;"("tau"=w720, "u0"=w740, "u1"=w733, "y1"=w732, "T"=0.001 ("input variable"), "a"=0.0 ("input variable"), "b"=1.0 ("input variable")) -> ("y0"=w450:dbl)
        n434 = feedback-in #37(w449) -> ()
        n435 = feedback-in #38(w451) -> ()
        n436 = feedback-in #39(w450) -> ()
        n437 = formula code="float W12,W123;\nif (abs(W1) > abs(W2))\nW12=W2;\nelse\nW12=W1;\n\nif (abs(W12) > abs(W3))\nW123= W3;\nelse\nW123=W12;\n\nMinW=W123;"("W1"=w451, "W2"=w450, "W3"=w449) -> ("MinW"=w439:dbl)
        "Vel_Robot" <- w439
        n438 = Subtract(x=w487, y=w439) -> (x-y=w533:dbl)
        n439 = Absolute Value(x=w439) -> (abs(x)=w489:dbl)
        n440 = Multiply(x=w533, y="Ki_V_cont") -> (x*y=w521:dbl)
        n441 = Greater?(x=w489, y=w490) -> (0:w480:bool)
        n442 = Multiply(x="Kp_V_cont 2", y=w533) -> (x*y=w517:dbl)
        "Kp_y" <- w517
        n443 = Add(x=w521, y=w519) -> (x+y=w520:dbl)
        n444 = Compound Arithmetic op=AND ("복합 연산")(w502, w480, FALSE ("값")) -> (w527:bool)
        n445 = formula code="y0=T*u+y1;"("u"=w520, "T"=0.001 ("입력 변수"), "y1"=w691) -> ("y0"=w678:dbl)
        "Ki_y" <- w678
        n446 = Not(x=w527) -> (.not. x?=w531:bool)
        n447 = Select(t=w532, s=w531, f=w487) -> (s? t:f=w530:dbl)
        n448 = Divide(x=w530, y=0.125) -> (x/y=w526:dbl)
        n449 = Select(t=w526, s=w380, f=0.0) -> (s? t:f=w528:dbl)
        n450 = Select(t=w525, s=w344, f=w528) -> (s? t:f=w589:dbl)
        n451 = feedback-in #33(w678) -> ()
        n452 = Add(x=w678, y=w517) -> (x+y=w488:dbl)
        n453 = formula code="if (u >= lim)\ny0=lim;\nelse if (u <= -lim)\ny0=-lim;\nelse\ny0=u;"("u"=w488, "lim"="ylimit") -> ("y0"=w524:dbl)
        "y*(Ki+Kp)" <- w524
        n454 = Subtract(x=w488, y=w524) -> (x-y=w523:dbl)
        "Wind_E" <- w523
        n455 = Multiply(x=w523, y="K_antiwind") -> (x*y=w516:dbl)
        n456 = Select(t=w516, s="Anti_wind", f=0.0) -> (s? t:f=w514:dbl)
        n457 = feedback-in #32(w514) -> ()
        n458 = Add(x="(1+y)_change", y=w524) -> (x+y=w680:dbl)
        n459 = Multiply(x=w680, y=w439) -> (x*y=w471:dbl)
        "V+yV" <- w471
        n460 = Absolute Value(x=w439) -> (abs(x)=w698:dbl)
        n461 = Greater?(x=w698, y="Vel_treshold") -> (0:w699:bool)
        n462 = Bundle("y0"=w452, "y0"=w454, "y0"=w453, "MinW"=w439) -> ()  [unwired: 1 in, 1 out]
        n463 = Compound Arithmetic op=AND ("복합 연산")(w569, w572, w531) -> (w588:bool)
        n464 = Multiply(x=w524, y=w679) -> (x*y=w687:dbl)
        n465 = Add(x=w439, y=w687) -> (x+y=w470:dbl)
        "V+yS" <- w470
        n466 = Select(t=w471, s=w699, f=w470) -> (s? t:f=w469:dbl)
        "VwRef" <- w469
        n467 = Select(t=w469, s=w502, f=0.0) -> (s? t:f=w507:dbl)
        n468 = Select(t=w507, s="No SRC(off)", f=w484) -> (s? t:f=w504:dbl)
        n469 = Divide(x=w504, y=0.125) -> (x/y=w505:dbl)
        n470 = case shown="거짓" w588 {
          tunnel: [w1207 w1208] -> w473
          tunnel: [w1207 w1208] -> w539
          tunnel: w505 -> [_ w1208]
          tunnel: [w1206 w1208] -> w538
          tunnel: w526 -> [w1207 _]
          tunnel: w589 -> [w1206 _]
          frame False {
          }
          frame True {
          }
        }
        "Ome_ref" <- w473
        n471 = feedback #56(0.0) -> (w1064:dbl)
        n472 = feedback-in #56(w1005) -> ()
        n473 = feedback #57(0.0) -> (w1093:dbl)
        n474 = Divide(x=w439, y=0.125) -> ()  [unwired: 1 out]
        n475 = Bundle(w451, w450, w449) -> (w447:cluster{dbl, dbl, dbl})  [unwired: 1 in]
        n476 = Or(x="From_SBC_DOB", y="YawConton") -> (x .or. y?=w630:bool)
        n477 = feedback #58(w878) -> (w995:dbl)
        n478 = case shown="참" w997 {
          tunnel: w412 -> [w1496 _]
          tunnel: [w1496 w1497] -> w877
          tunnel: w995 -> [_ w1497]
          frame False {
          }
          frame True {
          }
        }
        n479 = feedback-in #58(w877) -> ()
        n480 = Divide(x=w447, y=0.125) -> (x/y=w446:cluster{dbl, dbl, dbl})
        n481 = Select(t=w630, s=w621, f=FALSE) -> (s? t:f=w628:bool)
        n482 = Boolean To (0,1)(Boolean=w628) -> (0, 1=w1098:i16)
        n483 = Multiply(x=w1098, y=w1093) -> (x*y=w930:dbl)
        "DOB FB" <- w930
        n484 = feedback #59(0.0) -> (w559:dbl)
        n485 = feedback #60(0.0) -> (w567:dbl)
        n486 = Greater?(x=w700, y=300000) -> (0:w892:bool)
        n487 = Greater?(x=w700, y=210000) -> (0:w881:bool)
        n488 = Greater?(x=w700, y=270000) -> (0:w889:bool)
        n489 = Greater?(x=w700, y=240000) -> (0:w884:bool)
        n490 = Multiply(x="gy_offset_remover cutoff", y=6.283185307179586) -> (x*y=w1069:dbl)
        n491 = feedback #61(0.0) -> (w554:dbl)
        n492 = Subtract(x=w876, y=w877) -> (x-y=w875:dbl)
        n493 = Subtract(x=w327, y=w876) -> (x-y=w874:dbl)
        n494 = Subtract(x=w328, y=w327) -> (x-y=w326:dbl)
        n495 = Reciprocal(x=w1069) -> (1/x=w1056:dbl)
        n496 = Select(t=w445, s="Ome_FB_Ratelimit(off)", f=w446) -> (s? t:f=w444:cluster{"y0":dbl, "y0":dbl, "y0":dbl})
        n497 = Compound Arithmetic op=ADD(w875, w874, w326) -> (w873:dbl)
        n498 = Divide(x=w873, y=3.0) -> (x/y=w871:dbl)
        n499 = feedback #62(w878) -> (w893:dbl)
        n500 = case shown="참" w892 {
          tunnel: w412 -> [w1445 _]
          tunnel: [w1445 w1446] -> w894
          tunnel: w893 -> [_ w1446]
          frame False {
          }
          frame True {
          }
        }
        n501 = feedback-in #62(w894) -> ()
        n502 = feedback #63(w878) -> (w880:dbl)
        n503 = case shown="참" w881 {
          tunnel: w412 -> [w1451 _]
          tunnel: [w1451 w1452] -> w879
          tunnel: w880 -> [_ w1452]
          frame False {
          }
          frame True {
          }
        }
        n504 = feedback-in #63(w879) -> ()
        n505 = feedback #64(w878) -> (w888:dbl)
        n506 = case shown="참" w889 {
          tunnel: w412 -> [w1447 _]
          tunnel: [w1447 w1448] -> w887
          tunnel: w888 -> [_ w1448]
          frame False {
          }
          frame True {
          }
        }
        n507 = feedback-in #64(w887) -> ()
        n508 = feedback #65(w878) -> (w885:dbl)
        n509 = case shown="참" w884 {
          tunnel: w412 -> [w1449 _]
          tunnel: [w1449 w1450] -> w886
          tunnel: w885 -> [_ w1450]
          frame False {
          }
          frame True {
          }
        }
        n510 = feedback-in #65(w886) -> ()
        n511 = feedback #66(0.0) -> (w1068:dbl)
        n512 = formula code="float F,A,B,C,y0;\nF=2*tau+T;\nA=(2*a+b*T)/F;\nB=(b*T-2*a)/F;\nC=(2*tau-T)/F;\ny0=A*u0+B*u1+C*y1;"("tau"=w1056, "u0"=w1005, "u1"=w1064, "y1"=w1068, "T"=0.001 ("input variable"), "a"=0.0 ("input variable"), "b"=1.0 ("input variable")) -> ("y0"=w1041:dbl)
        n513 = feedback-in #66(w1041) -> ()
        n514 = Divide(x="J_FF_R_wh", y="Kt_longi") -> (x/y=w644:dbl)
        n515 = Multiply(x="right wheel FF_cut 2", y=6.283185307179586) -> (x*y=w660:dbl)
        n516 = feedback #67(0.0 ("gy_z[]")) -> (w664:dbl)
        n517 = feedback-in #67(w538) -> ()
        n518 = Multiply(x="right wheel FF_cut 2", y=6.283185307179586) -> (x*y=w667:dbl)
        n519 = Unbundle(w444) -> ("y0"=w458:dbl, "y0"=w457:dbl, "y0"=w463:dbl)
        "Ome_rear" <- w463
        "Ome_L" <- w457
        "Ome_R" <- w458
        n520 = Subtract(x=w473, y=w458) -> (x-y=w550:dbl)
        n521 = Subtract(x=w539, y=w457) -> (x-y=w551:dbl)
        n522 = Subtract(x=w538, y=w463) -> (x-y=w563:dbl)
        n523 = Multiply(x=w550, y="Kp_wheelomega_Cont") -> (x*y=w549:dbl)
        n524 = Multiply(x="Kp_wheelomega_Cont", y=w563) -> (x*y=w564:dbl)
        n525 = Multiply(x=w551, y="Ki_wheel\nomega_cont") -> (x*y=w560:dbl)
        n526 = Multiply(x=w551, y="Kp_wheelomega_Cont") -> (x*y=w557:dbl)
        n527 = Multiply(x=w550, y="Ki_wheel\nomega_cont") -> (x*y=w553:dbl)
        n528 = Multiply(x="Ki_wheel\nomega_cont", y=w563) -> (x*y=w562:dbl)
        n529 = formula code="y0=0.001*u+y1;"("u"=w560, "y1"=w559) -> ("y0"=w558:dbl)
        n530 = formula code="y0=0.001*u+y1;"("u"=w553, "y1"=w554) -> ("y0"=w472:dbl)
        n531 = formula code="y0=0.001*u+y1;"("u"=w562, "y1"=w567) -> ("y0"=w565:dbl)
        n532 = feedback-in #59(w558) -> ()
        n533 = feedback-in #60(w565) -> ()
        n534 = feedback-in #61(w472) -> ()
        n535 = Add(x=w564, y=w565) -> (x+y=w566:dbl)
        n536 = Add(x=w558, y=w557) -> (x+y=w556:dbl)
        n537 = Add(x=w472, y=w549) -> (x+y=w548:dbl)
        n538 = feedback #68(0.0 ("gy_z[]")) -> (w671:dbl)
        n539 = feedback-in #68(w473) -> ()
        n540 = Reciprocal(x=w660) -> (1/x=w662:dbl)
        n541 = Reciprocal(x=w667) -> (1/x=w669:dbl)
        n542 = Greater?(x=w700, y=91000) -> ()  [unwired: 1 out]
        n543 = Greater?(x=w700, y=40000) -> (0:w1052:bool)
        n544 = Greater?(x=w700, y=35000) -> (0:w1057:bool)
        n545 = Greater?(x=w700, y=45000) -> (0:w1051:bool)
        n546 = Greater?(x=w700, y=61000) -> (0:w501:bool)
        "Readyon" <- w501
        n547 = case shown="참" w501 {
          tunnel: [180 w1494] -> w976
          tunnel: w412 -> [_ w1490]
          tunnel: w700 -> [_ w1492]
          tunnel: w871 -> [_ w1489]
          frame False {
          }
          frame True {
            n548 = Divide(x=w1489, y=10000) -> (x/y=w1493:dbl)
            n549 = Multiply(x=w1493, y=w1492) -> (x*y=w1491:dbl)
            n550 = Subtract(x=w1490, y=w1491) -> (x-y=w1494:dbl)
          }
        }
        n551 = Divide(x="B_FF_R_wh", y="Kt_longi") -> (x/y=w645:dbl)
        n552 = feedback #69(0.0 ("gy_z[]")) -> (w663:dbl)
        n553 = formula code="float F,A,B,C,y0;\nF=2*tau+T;\nA=(2*a+b*T)/F;\nB=(b*T-2*a)/F;\nC=(2*tau-T)/F;\ny0=A*u0+B*u1+C*y1;"("tau"=w662, "u0"=w538, "u1"=w664, "y1"=w663, "T"=0.001 ("input variable"), "a"=w644, "b"=w645) -> ("y0"=w537:dbl)
        n554 = Add(x=w537, y=w566) -> (x+y=w646:dbl)
        n555 = feedback-in #69(w537) -> ()
        n556 = feedback #70(0.0 ("gy_z[]")) -> (w670:dbl)
        n557 = formula code="float F,A,B,C,y0;\nF=2*tau+T;\nA=(2*a+b*T)/F;\nB=(b*T-2*a)/F;\nC=(2*tau-T)/F;\ny0=A*u0+B*u1+C*y1;"("tau"=w669, "u0"=w473, "u1"=w671, "y1"=w670, "T"=0.001 ("input variable"), "a"=w644, "b"=w645) -> ("y0"=w464:dbl)
        n558 = Select(t=w464, s="FFOn", f=0.0) -> (s? t:f=w460:dbl)
        n559 = Add(x=w548, y=w460) -> (x+y=w459:dbl)
        n560 = Select(t=w464, s="FFOn", f=0.0) -> (s? t:f=w465:dbl)
        n561 = Add(x=w556, y=w465) -> (x+y=w440:dbl)
        n562 = feedback-in #70(w464) -> ()
        n563 = feedback #71(w1048) -> (w1045:dbl)
        n564 = case shown="거짓" w1057 {
          tunnel: w1041 -> [w1504 _]
          tunnel: [w1504 w1505] -> w1055
          tunnel: w1045 -> [_ w1505]
          frame False {
          }
          frame True {
          }
        }
        n565 = feedback-in #71(w1055) -> ()
        n566 = feedback #72(w1048) -> (w1047:dbl)
        n567 = case shown="거짓" w1051 {
          tunnel: w1041 -> [w1500 _]
          tunnel: [w1500 w1501] -> w1049
          tunnel: w1047 -> [_ w1501]
          frame False {
          }
          frame True {
          }
        }
        n568 = feedback-in #72(w1049) -> ()
        n569 = feedback #73(w1048) -> (w1046:dbl)
        n570 = case shown="거짓" w1052 {
          tunnel: w1041 -> [w1502 _]
          tunnel: [w1502 w1503] -> w1050
          tunnel: w1046 -> [_ w1503]
          frame False {
          }
          frame True {
          }
        }
        n571 = feedback-in #73(w1050) -> ()
        n572 = Compound Arithmetic op=ADD(w1047, w1046, w1045) -> (w1044:dbl)
        n573 = Divide(x=w1044, y=3.0) -> (x/y=w1024:dbl)
        n574 = Subtract(x=w1005, y=w1024) -> (x-y=w1020:dbl)
        n575 = formula code="float rate;\nrate=gy-gy_r1;\nif (rate > limit)\ngy_ratelimit=gy_r1+limit;\nelse if (rate < -limit)\ngy_ratelimit=gy_r1+(-limit);\nelse\ngy_ratelimit=gy;"("gy"=w1020, "gy_r1"=w1040, "limit"="yaw_ratelimit") -> ("gy_ratelimit"=w1023:dbl)
        n576 = feedback-in #42(w1023) -> ()
        n577 = feedback-in #44(w1023) -> ()
        n578 = formula code="float F,A,B,C,y0;\nF=2*tau+T;\nA=(2*a+b*T)/F;\nB=(b*T-2*a)/F;\nC=(2*tau-T)/F;\ny0=A*u0+B*u1+C*y1;"("tau"=w1035, "u0"=w1023, "u1"=w1033, "y1"=w1038, "T"=0.001 ("input variable"), "a"=0.0 ("input variable"), "b"=1.0 ("input variable")) -> ("y0"=w1028:dbl)
        n579 = feedback-in #55(w1028) -> ()
        n580 = formula code="float band_ratelim;\n\nif (gy_ratelim < gy_band && gy_ratelim > -gy_band)\nband_ratelim=0;\nelse\nband_ratelim=gy_ratelim;"("gy_ratelim"=w1028, "gy_band"="ratelimit band") -> ("band_ratelim"=w936:dbl)
        n581 = Multiply(x="gyro scale", y=w936) -> (x*y=w493:dbl)
        "GyroFB" <- w493
        n582 = Subtract(x=w978, y=w493) -> (x-y=w1081:dbl)
        n583 = feedback-in #18(w1081) -> ()
        n584 = formula code="float F,A,B,C,ykd,ykp,y0;\nF=2*tau+T;\nA=(2*Kd_rot)/F;\nB=(-2*Kd_rot)/F;\nC=(2*tau-T)/F;\nykd=A*u0+B*u1+C*y1;\nykp=Kp_rot*u0;\ny0=ykp+ykd;"("tau"=w1084, "u0"=w1081, "u1"=w1082, "y1"=w1077, "T"=0.001 ("input variable"), "Kp_rot"="Kp_rot 2", "Kd_rot"="Kd_rot 3") -> ("y0"=w1074:dbl)
        n585 = feedback-in #23(w1074) -> ()
        n586 = Select(t=w1074, s=w955, f=0.0) -> (s? t:f=w1060:dbl)
        "RotFB" <- w1060
        n587 = Add(x=w1076, y=w1060) -> (x+y=w931:dbl)
        n588 = Subtract(x=w931, y=w930) -> (x-y=w649:dbl)
        n589 = Negate(x=w649) -> (-x=w653:dbl)
        n590 = Select(t=w649, s=w652, f=w653) -> (s? t:f=w335:dbl)
        "Tq ang in" <- w335
        n591 = feedback-in #40(w649) -> ()
        n592 = feedback-in #41(w493) -> ()
        n593 = formula code="float F,A,B,C,y0;\nF=2*tau+T;\nA=(2*a+b*T)/F;\nB=(b*T-2*a)/F;\nC=(2*tau-T)/F;\ny0=A*u0+B*u1+C*y1;"("tau"=w1114, "u0"=w493, "u1"=w1108, "y1"=w1107, "T"=w1109, "a"=w1102, "b"=w1101) -> ("y0"=w1097:dbl)
        n594 = formula code="float F,A,B,C,y0;\nF=2*tau+T;\nA=(2*a+b*T)/F;\nB=(b*T-2*a)/F;\nC=(2*tau-T)/F;\ny0=A*u0+B*u1+C*y1;"("tau"=w1114, "u0"=w649, "u1"=w1111, "y1"=w1110, "T"=w1109, "a"=0.0 ("input variable"), "b"=1.0 ("input variable")) -> ("y0"=w1100:dbl)
        n595 = formula code="if (u >= lim*10/10)\ny0=lim*10/10;\nelse if (u <= -lim*10/10)\ny0=-lim*10/10;\nelse\ny0=u;"("u"=w335, "lim"="Steeing_Tq*_limit") -> ("y0"=w475:dbl)
        n596 = feedback-in #48(w1100) -> ()
        n597 = feedback-in #49(w1097) -> ()
        n598 = Subtract(x=w1097, y=w1100) -> (x-y=w1099:dbl)
        n599 = feedback-in #57(w1099) -> ()
        n600 = formula code="if (ang > 360)\nang1=ang-360;\nelse\nang1=ang;"("ang"=w976) -> ("ang1"=→"ang_bias remover":dbl)
        n601 = formula code="if (u >= lim*1)\ny0=lim*1;\nelse if (u <= -lim*1)\ny0=-lim*1;\nelse\ny0=u;"("u"=w459, "lim"="Tq limit[V]") -> ("y0"=w462:dbl)
        n602 = formula code="if (u >= lim*1)\ny0=lim*1;\nelse if (u <= -lim*1)\ny0=-lim*1;\nelse\ny0=u;"("u"=w440, "lim"="Tq limit[V]") -> ("y0"=w461:dbl)
        n603 = formula code="if (u >= lim*1)\ny0=lim*1;\nelse if (u <= -lim*1)\ny0=-lim*1;\nelse\ny0=u;"("u"=w646, "lim"="Tq limit[V]") -> ("y0"=w702:dbl)
        n604 = Bundle(w459, w440, "MinW"=w439) -> (→"Tq_vel":cluster{dbl, dbl, "MinW":dbl})  [unwired: 1 in]
        n605 = Not(x=w502) -> (.not. x?=w818:bool)
        n606 = Greater?(x=w439, y=1.0) -> (0:w827:bool)
        n607 = And(x=w827, y=w818) -> (x .and. y?=w823:bool)
        n608 = feedback #74(0.0) -> (w824:dbl)
        n609 = case shown="거짓" w823 {
          tunnel: w377 -> [w1435 _]
          tunnel: [w1435 w1436] -> w825
          tunnel: w824 -> [_ w1436]
          frame False {
          }
          frame True {
          }
        }
        n610 = feedback-in #74(w825) -> ()
        n611 = Not(x=w383) -> (.not. x?=w606:bool)
        n612 = Subtract(x=w377, y=w825) -> (x-y=w809:dbl)
        n613 = Less?(x=w809, y=0.01) -> (x < y?=w813:bool)
        n614 = Greater?(x=w809, y=0.0) -> (0:w812:bool)
        n615 = And(x=w812, y=w813) -> (x .and. y?=w808:bool)
        n616 = local read "Time_int"() -> (w433:i32)
        n617 = local read "DriveMODE"() -> (w427:dbl)
        n618 = Divide(x=w438, y="scale_Ang_steer/ 2") -> (x/y=w477:dbl)
        n619 = Divide(x=w433, y=1000) -> (x/y=w428:dbl)
        n620 = Divide(x=w475, y="scale_Ang_steer/") -> (x/y=w474:dbl)
        n621 = Select(t=w474, s=w606, f=w477) -> (s? t:f=w476:dbl)
        "Tq_Steer" <- w476
        n622 = feedback #75(0.0) -> (w430:dbl)
        n623 = feedback #76(0.0) -> (w817:dbl)
        n624 = case shown="거짓" w808 {
          tunnel: w377 -> [_ w1434]
          tunnel: [w1433 w1434] -> w816
          tunnel: w817 -> [w1433 _]
          frame False {
          }
          frame True {
          }
        }
        n625 = feedback-in #76(w816) -> ()
        n626 = Equal?(x=w427, y=4.0) -> (x = y?=w425:bool)
        n627 = Or(x=w425, y="SaveReset") -> (x .or. y?=w423:bool)
        n628 = case shown="거짓" w423 {
          tunnel: w428 -> [_ w1162]
          tunnel: [w1161 w1162] -> w429
          tunnel: w430 -> [w1161 _]
          frame False {
          }
          frame True {
          }
        }
        n629 = feedback-in #75(w429) -> ()
        n630 = Add(x=w476, y=2.5) -> (x+y=w706:dbl)
        n631 = Subtract(x=w428, y=w429) -> (x-y=w414:dbl)
        n632 = Subtract(x=w377, y=w816) -> (x-y=w814:dbl)
        n633 = formula code="if (u >= 5)\ny0=5;\nelse if (u <= 0)\ny0=0;\nelse\ny0=u;"("u"=w706) -> ("y0"=w705:dbl)
        n634 = Greater?(x=w414, y=0.1) -> (0:w420:bool)
        n635 = Less?(x=w414, y=0.12) -> (x < y?=w419:bool)
        n636 = Greater?(x=w414, y=0.2) -> (0:w417:bool)
        n637 = Less?(x=w414, y=0.22) -> (x < y?=w418:bool)
        n638 = Greater?(x=w814, y=0.0) -> (0:w820:bool)
        n639 = Less?(x=w814, y=10.0) -> (x < y?=w819:bool)
        n640 = And(x=w420, y=w419) -> (x .and. y?=→"write":bool)
        n641 = And(x=w417, y=w418) -> (x .and. y?=→"reset":bool)
        n642 = And(x=w820, y=w819) -> (x .and. y?=w806:bool)
        n643 = Greater?(x=w439, y=0.1) -> (0:w805:bool)
        n644 = And(x=w805, y=w806) -> (x .and. y?=w546:bool)
        n645 = Not(x=w546) -> (.not. x?=w634:bool)
        n646 = Select(t=w702, s=w634, f=0.0) -> (s? t:f=w703:dbl)
        n647 = Divide(x=w703, y="Rear_scale") -> (x/y=w585:dbl)
        "Tq_cmd_Rear" <- w585
        n648 = Add(x=w585, y=2.5) -> (x+y=w586:dbl)
        n649 = formula code="if (u >= 5)\ny0=5;\nelse if (u <= 0)\ny0=0;\nelse\ny0=u;"("u"=w586) -> ("y0"=w584:dbl)
        n650 = case shown="참" w546 {
          tunnel: [0.0 ("f") "Tq_stop"] -> w648
          frame False {
          }
          frame True {
          }
        }
        n651 = Select(t=w461, s=w634, f=w648) -> (s? t:f=w486:dbl)
        "Tq_cmd_L" <- w486
        n652 = Select(t=w462, s=w634, f=w648) -> (s? t:f=w485:dbl)
        "Tq_cmd_R" <- w485
        n653 = Negate(x=w486) -> (-x=w708:dbl)
        n654 = xnode "Analog output (1 sample)"("C/AO0 (AO0)"=w485, "C/AO1 (AO1)"=w708, "rearDriving (A/AO0 (Pin 2))"=w584, "RearSteer (A/AO1 (Pin 4))"=w705) -> ()  [unwired: 1 in, 1 out]
        n655 = node-c288() -> ()  [unwired: 1 in, 1 out]
        "Time_int" <- w700
        "Driving" <- "Drive_Enable"
      }
      n656 = call <vilib>:"Simple Error Handler.vi"("error in (no error)"=w147) -> ("error out"=w156:errorcluster)  [unwired: 4 in, 4 out]
      n657 = call <vilib>:"Reset myRIO.vi"("error in (no error)"=w156) -> ()  [unwired: 10 in, 1 out]
      n658 = node-c288(w130) -> ()  [unwired: 1 out]
      n659 = while {
        i -> [w214]
        stop <- "file create" stop-if-true
        n660 = Format Date/Time String(time format string (%c)="%Y%m%d_%H%M%S%3u") -> (date/time string=w212:string)  [unwired: 2 in]
        n661 = Strip Path(path=path "U:/Users") -> (stripped path=w207:path)  [unwired: 1 out]
        n662 = Concatenate Strings(w212, ".csv" ("string")) -> (w210:string)
        n663 = while {
          i -> [w217]
          stop <- w216 stop-if-true
          n664 = local read "reset"() -> (w216:bool)
          "Numeric Control" <- w217
        }
        n665 = Build Path(base path=w207, name or relative path=w210) -> (appended path=w209:path)
        n666 = Open/Create/Replace File(file path (use dialog)=w209, operation (0:open)=T15."create") -> (refnum out=w205:refnum<file>)  [unwired: 4 in, 2 out]
        n667 = while {
          tunnel: w205 -> [w265]
          tunnel: [w264] -> w204
          i -> [w272]
          stop <- w243 stop-if-true
          n668 = Wait Until Next ms Multiple(millisecond multiple=u32 10 ("ms 배수")) -> ()  [unwired: 1 out]
          n669 = local read "write"() -> (w243:bool)
          n670 = local read "DEn"() -> (w227:bool)
          n671 = local read "StEn"() -> (w226:bool)
          n672 = xnode "Accelerometer"() -> ("X-Axis"=w242:dbl, "Y-Axis"=w241:dbl)  [unwired: 1 in, 1 out]
          n673 = Boolean To (0,1)(Boolean=w226) -> (0, 1=w222:i16)
          n674 = Boolean To (0,1)(Boolean=w227) -> (0, 1=w224:i16)
          n675 = local read "RearEn"() -> (w218:i16)
          n676 = Multiply(x=w224, y=1.0) -> (x*y=w220:dbl)
          n677 = Multiply(x=w222, y=1.0) -> (x*y=w219:dbl)
          n678 = local read "Ome_R"() -> (w251:dbl)
          n679 = Multiply(x=w218, y=1.0) -> (x*y=w221:dbl)
          n680 = local read "delta_ang_memo"() -> (w253:dbl)
          n681 = local read "AngNowCmd"() -> (w255:dbl)
          n682 = local read "AngNowFB"() -> (w254:dbl)
          n683 = local read "DriveMode"() -> (w245:dbl)
          n684 = local read "YRRefOn"() -> (w234:dbl)
          n685 = local read "Tq_cmd_L"() -> (w239:dbl)
          n686 = local read "Tq_cmd_R"() -> (w240:dbl)
          n687 = local read "Vel_Robot"() -> (w249:dbl)
          n688 = local read "Tq_cmd_Rear"() -> (w238:dbl)
          n689 = local read "DOB FB"() -> (w232:dbl)
          n690 = local read "Ome_ref"() -> (w250:dbl)
          n691 = local read "V+yS"() -> (w244:dbl)
          n692 = local read "nowphi"() -> (w257:dbl)
          n693 = local read "Ome_L"() -> (w252:dbl)
          n694 = local read "VwRef"() -> (w261:dbl)
          n695 = Format Date/Time String(time format string (%c)="%H%M%S%3u") -> (date/time string=w269:string)  [unwired: 2 in]
          n696 = local read "l_rear"() -> (w247:dbl)
          n697 = local read "V+yV"() -> (w260:dbl)
          n698 = local read "angle"() -> (w256:dbl)
          n699 = local read "Tq_Steer"() -> (w237:dbl)
          n700 = local read "Kp_y"() -> (w258:dbl)
          n701 = local read "Ki_y"() -> (w259:dbl)
          n702 = local read "YRRef"() -> (w233:dbl)
          n703 = local read "Vref"() -> (w248:dbl)
          n704 = local read "SteerAng"() -> (w235:dbl)
          n705 = local read "th_steer"() -> (w236:dbl)
          n706 = local read "ang_bias remover"() -> (w229:dbl)
          n707 = local read "RotFF"() -> (w231:dbl)
          n708 = local read "RotFB"() -> (w230:dbl)
          n709 = Bundle("l_rear"=w247, "Vref"=w248, "Vel_Robot"=w249, "Ome_ref"=w250, "Ome_R"=w251, "Ome_L"=w252, "VwRef"=w261, "V+yV"=w260, "V+yS"=w244, "Ki_y"=w259, "Kp_y"=w258, "nowphi"=w257, "angle"=w256, "AngNowCmd"=w255, "AngNowFB"=w254, "delta_ang_memo"=w253, "DriveMode"=w245, "X-Axis"=w242, "Y-Axis"=w241, "Tq_cmd_R"=w240, "Tq_cmd_L"=w239, "Tq_cmd_Rear"=w238, "Tq_Steer"=w237, "th_steer"=w236, "SteerAng"=w235, "YRRefOn"=w234, "YRRef"=w233, "DOB FB"=w232, "RotFF"=w231, "RotFB"=w230, "ang_bias remover"=w229, w221, w220, w219) -> (w246:T31)  [unwired: 1 in]
          n710 = Cluster To Array(cluster=w246) -> (array=w262:dbl[])
          n711 = Array To Spreadsheet String(array=w262, 3:"%f" ("format string")) -> (spreadsheet string=w266:string)  [unwired: 1 in]
          n712 = Concatenate Strings(w269, "\t", w266) -> (w271:string)
          n713 = Write to Text File(file (use dialog)=w265, text=w271) -> (refnum out=w264:refnum<file>)  [unwired: 2 in, 2 out]
          "data innter" <- w272
        }
        n714 = Close File(refnum=w204) -> ()  [unwired: 1 in, 2 out]
        "File create" <- w214
      }
    }
  }
